vi "Autonomous Independent.vi"() -> ()   [LabVIEW 2020]
doc: "This VI is called when autonomous begins, and will automatically be terminated when autonomous ends. You can carry out timed or sensor driven robot movement independently without needing to return to the caller."
uses:
  <vilib>/Rock Robotics/WPI/ThirdParty/Phoenix-LabVIEW/Motor Controller/Controls/CTRE_Phoenix_MotorControl_ControlMode.ctl
  <vilib>/Rock Robotics/WPI/Solenoid/WPI_SolenoidValue.ctl
  <vilib>/Rock Robotics/WPI/Utilities/WPI_GetSetVariantRefNum.vi
  <vilib>/Rock Robotics/Network Tables/NT Read String.vi
  <vilib>/Rock Robotics/Network Tables/NT Write Numeric Array.vi
  <vilib>/Rock Robotics/WPI/Solenoid/WPI_SolenoidSetEnum.vi
  <vilib>/Rock Robotics/Network Tables/NT Read Number.vi
panel:
  out "Ty 22":dbl
  out "Ty 21":dbl
  out "Ty 20":dbl
  out "Ty 19":dbl
  out "Ty 18":dbl
  out "Ty 17":dbl
  out "Orange Limit Pressed 10":bool
  out "Blue Limit Pressed 10":bool
  out "Ty 16":dbl
  out "Orange Limit Pressed 9":bool
  out "Blue Limit Pressed 9":bool
  out "Ty 15":dbl
  out "Intake 5":bool
  out "Elevate 5":bool
  out "Ty 14":dbl
  out "Ty 13":dbl
  out "Ty 12":dbl
  out "Ty 11":dbl
  out "Ty 10":dbl
  out "Ty 9":dbl
  out "Orange Limit Pressed 4":bool
  out "Blue Limit Pressed 4":bool
  out "Ty 4":dbl
  out "Orange Limit Pressed 3":bool
  out "Blue Limit Pressed 3":bool
  out "Ty 3":dbl
  out "Intake 2":bool
  out "Elevate 2":bool
  out "Intake":bool
  out "Elevate":bool
  out "Orange Limit Pressed":bool
  out "Blue Limit Pressed":bool
  out "Ty":dbl
  out "Orange Limit Pressed 2":bool
  out "Blue Limit Pressed 2":bool
  out "Ty 2":dbl
  out "Intake 3":bool
  out "Elevate 3":bool
  out "Orange Limit Pressed 5":bool
  out "Blue Limit Pressed 5":bool
  out "Ty 5":dbl
  out "Orange Limit Pressed 6":bool
  out "Blue Limit Pressed 6":bool
  out "Ty 6":dbl
  out "Intake 4":bool
  out "Elevate 4":bool
  out "Orange Limit Pressed 7":bool
  out "Blue Limit Pressed 7":bool
  out "Ty 7":dbl
  out "Orange Limit Pressed 8":bool
  out "Blue Limit Pressed 8":bool
  out "Ty 8":dbl
  # "Be sure to right-click and choose Data Operations>>Make Current Value default if you want to save the array values with the VI"
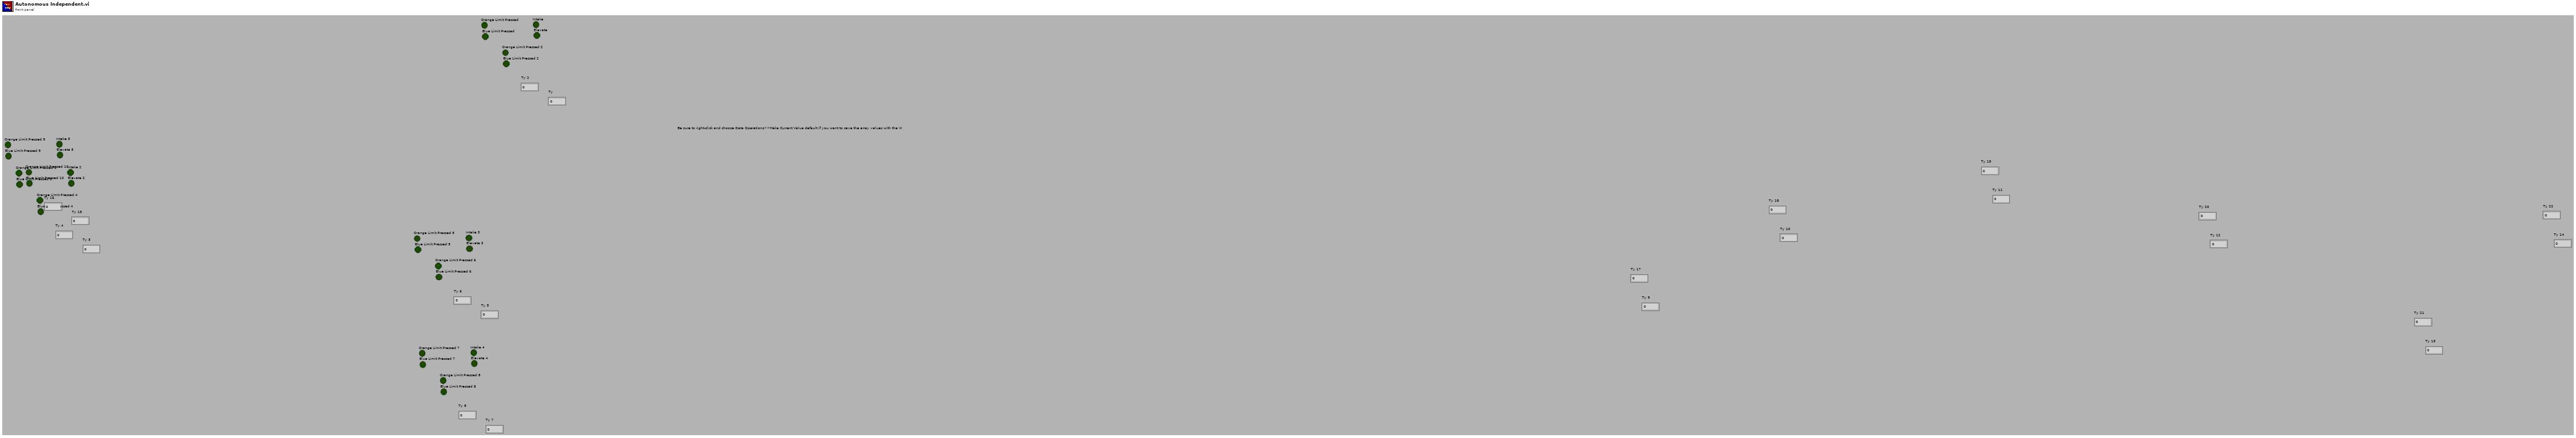
[diagram p1: front panel]
types:
  T1 = typedef "WPI_JoystickDevRef.ctl" = cluster{"Device":T2}
  T2 = typedef "WPI_JoystickDeviceEnum.ctl" = enum16{"USB 0", "USB 1", "USB 2", "USB 3", "USB 4", "USB 5"}
  T3 = typedef "WPI_SolenoidValue.ctl" = enum16{"Off", "On", "Forward", "Reverse"}
  T4 = typedef "WPI_SwitchDevRef.ctl" = cluster{"DevStatus":errorcluster, "DIO Channel":T5, "CntIndex":T6, "Normally Closed":bool}
  T5 = typedef "FPGA_DIOChannel.ctl" = enum8{"DIO 0", "DIO 1", "DIO 2", "DIO 3", "DIO 4", "DIO 5", "DIO 6", "DIO 7", "DIO 8", "DIO 9", "DIO MXP 0", "DIO MXP 1", "DIO MXP 2", "DIO MXP 3", "DIO MXP 4", "DIO MXP 5", "DIO MXP 6", "DIO MXP 7", "DIO MXP 8", "DIO MXP 9", "DIO MXP 10", "DIO MXP 11", "DIO MXP 12", "DIO MXP 13", "DIO MXP 14", "DIO MXP 15", "SPI Port CS1", "SPI Port CS2", "SPI Port CS3", "SPI Port MISO", "SPI Port MOSI", "Invalid"}
  T6 = typedef "FPGA_CounterCtrSystemIndex.ctl" = enum8{"Ctr 0", "Ctr 1", "Ctr 2", "Ctr 3", "Ctr 4", "Ctr 5", "Ctr 6", "Ctr 7", "Invalid"}
  T7 = typedef "WPI_SolenoidDevRef.ctl" = cluster{"DevStatus":errorcluster, "Pneumatics Control Module":u8, "Forward Solenoid Channel":T8, "Reverse Solenoid Channel":T8}
  T8 = typedef "WPI_SolenoidChannel.ctl" = enum8{"Solenoid 0", "Solenoid 1", "Solenoid 2", "Solenoid 3", "Solenoid 4", "Solenoid 5", "Solenoid 6", "Solenoid 7", "Solenoid 8", "Solenoid 9", "Solenoid 10", "Solenoid 11", "Solenoid 12", "Solenoid 13", "Solenoid 14", "Solenoid 15", "Invalid"}
  T9 = typedef "WPI_MotorControlDeviceRef.ctl" = cluster{"DeviceStatus":errorcluster, "Type":T10, "PWM":cluster{"PWM Channel":T11, "DeadBand":T12}, "CAN":cluster{"Device Number":u8, "SetOutput VI Ref":variant, "GetOutput VI Ref":variant, "Enable VI Ref":variant, "Disable VI Ref":variant, "Data":variant}, "Invert":bool, "DIO PWM":cluster{"PWM \"Enable\" Channel":T11, "DIOChannel":T5, "PWM Rate":dbl}}
  T10 = typedef "WPI_MotorControlType.ctl" = enum16{"PWM", "CAN", "DIO PWM"}
  T11 = typedef "FPGA_DIOPWMChannel.ctl" = enum8{"PWM 0", "PWM 1", "PWM 2", "PWM 3", "PWM 4", "PWM 5", "PWM 6", "PWM 7", "PWM 8", "PWM 9", "PWM MXP 0", "PWM MXP 1", "PWM MXP 2", "PWM MXP 3", "PWM MXP 4", "PWM MXP 5", "PWM MXP 6", "PWM MXP 7", "PWM MXP 8", "PWM MXP 9", "Invalid"}
  T12 = typedef "WPI_PWMDeadband.ctl" = cluster{"Name":string, "maxPositivePwm":i32, "minPositivePwm":i32, "centerPwm":i32, "maxNegativePwm":i32, "minNegativePwm":i32, "angularRange":u16}
  T13 = typedef "CTRE_Phoenix_MotorControl_ControlMode.ctl" = u16
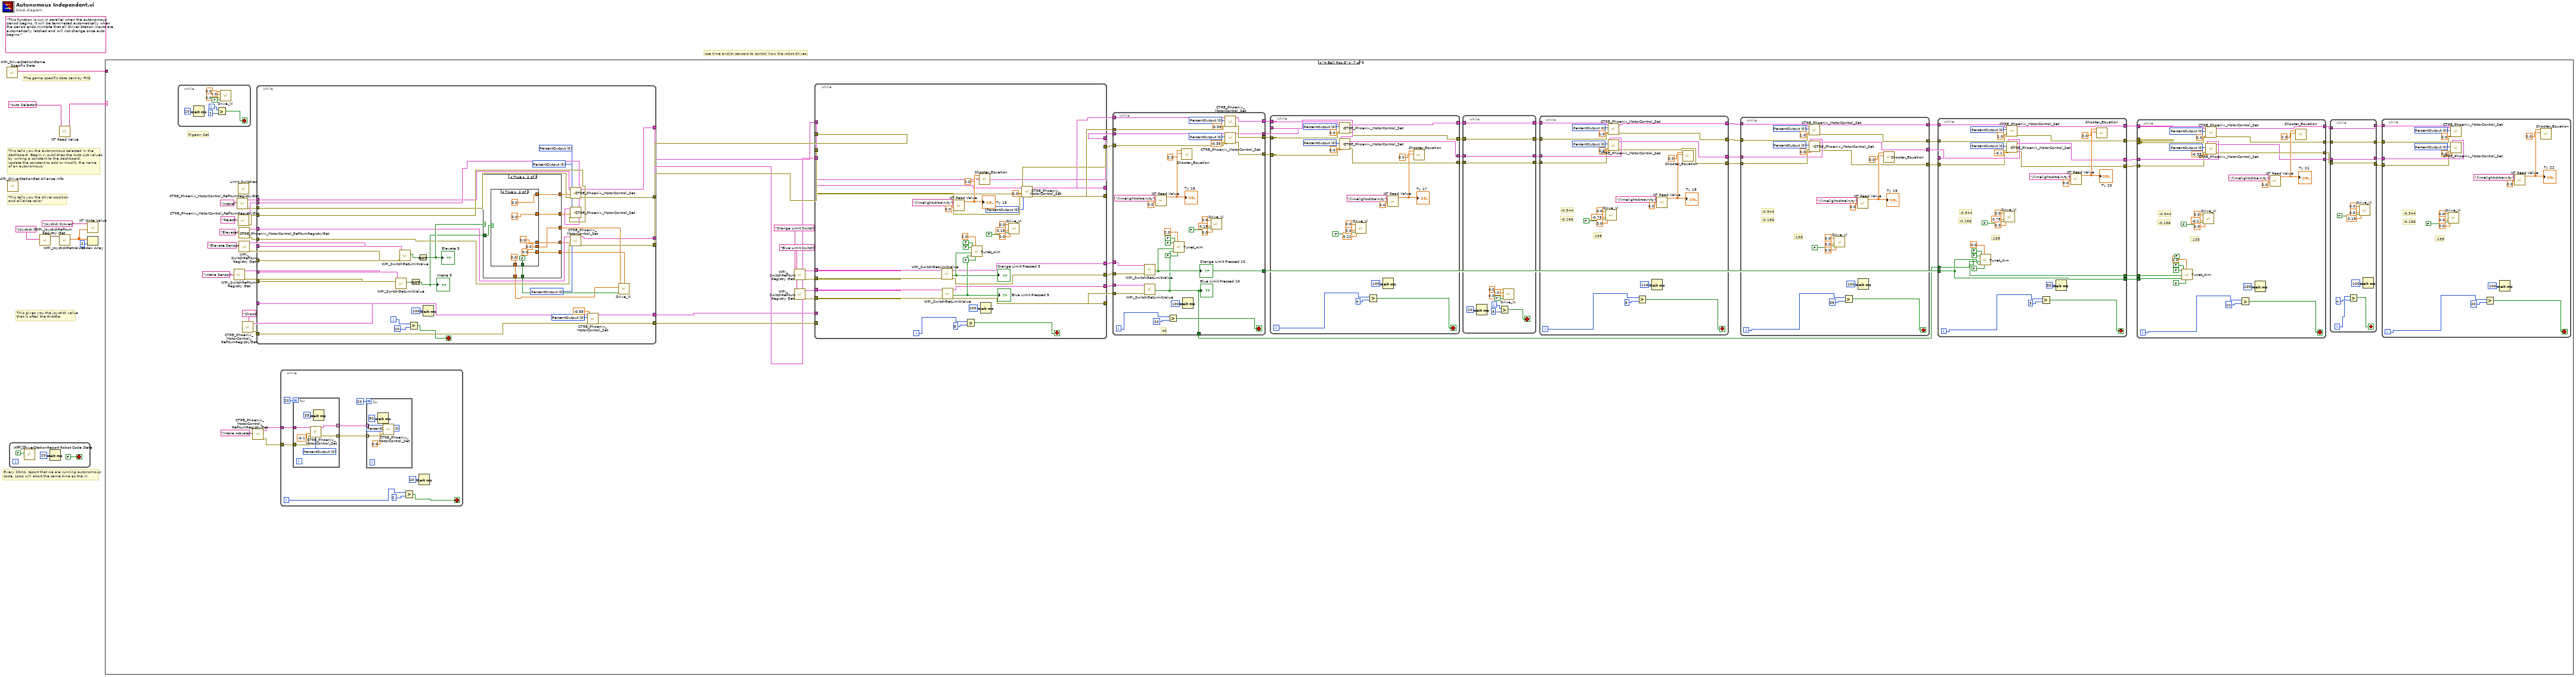
[diagram p0: block diagram]
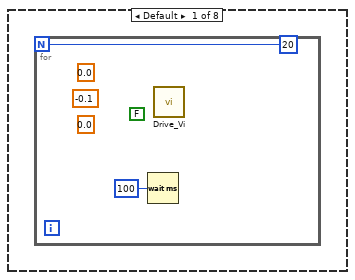
[diagram p2: hidden frame]
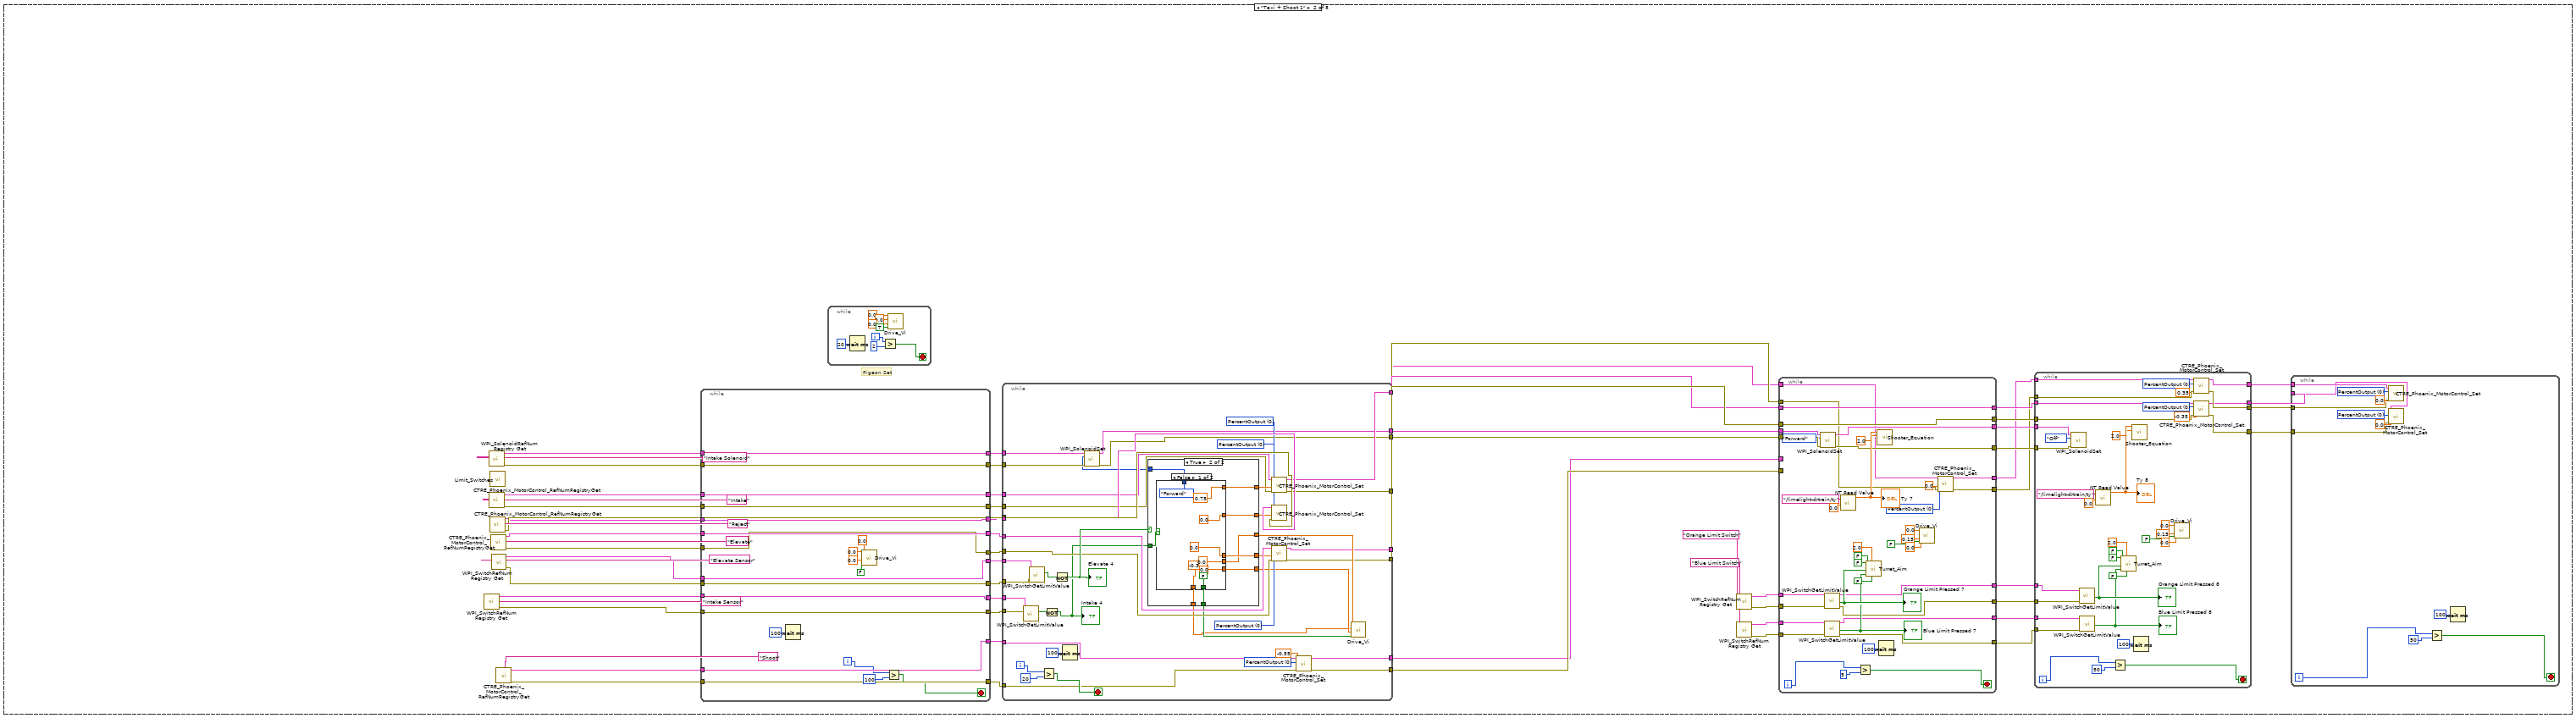
[diagram p3: hidden frame]
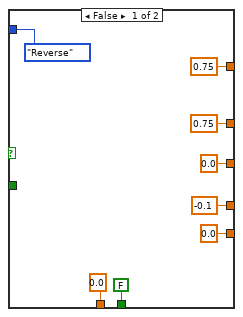
[diagram p4: hidden frame]
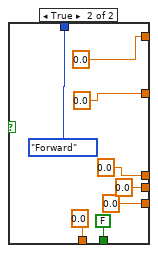
[diagram p5: hidden frame]
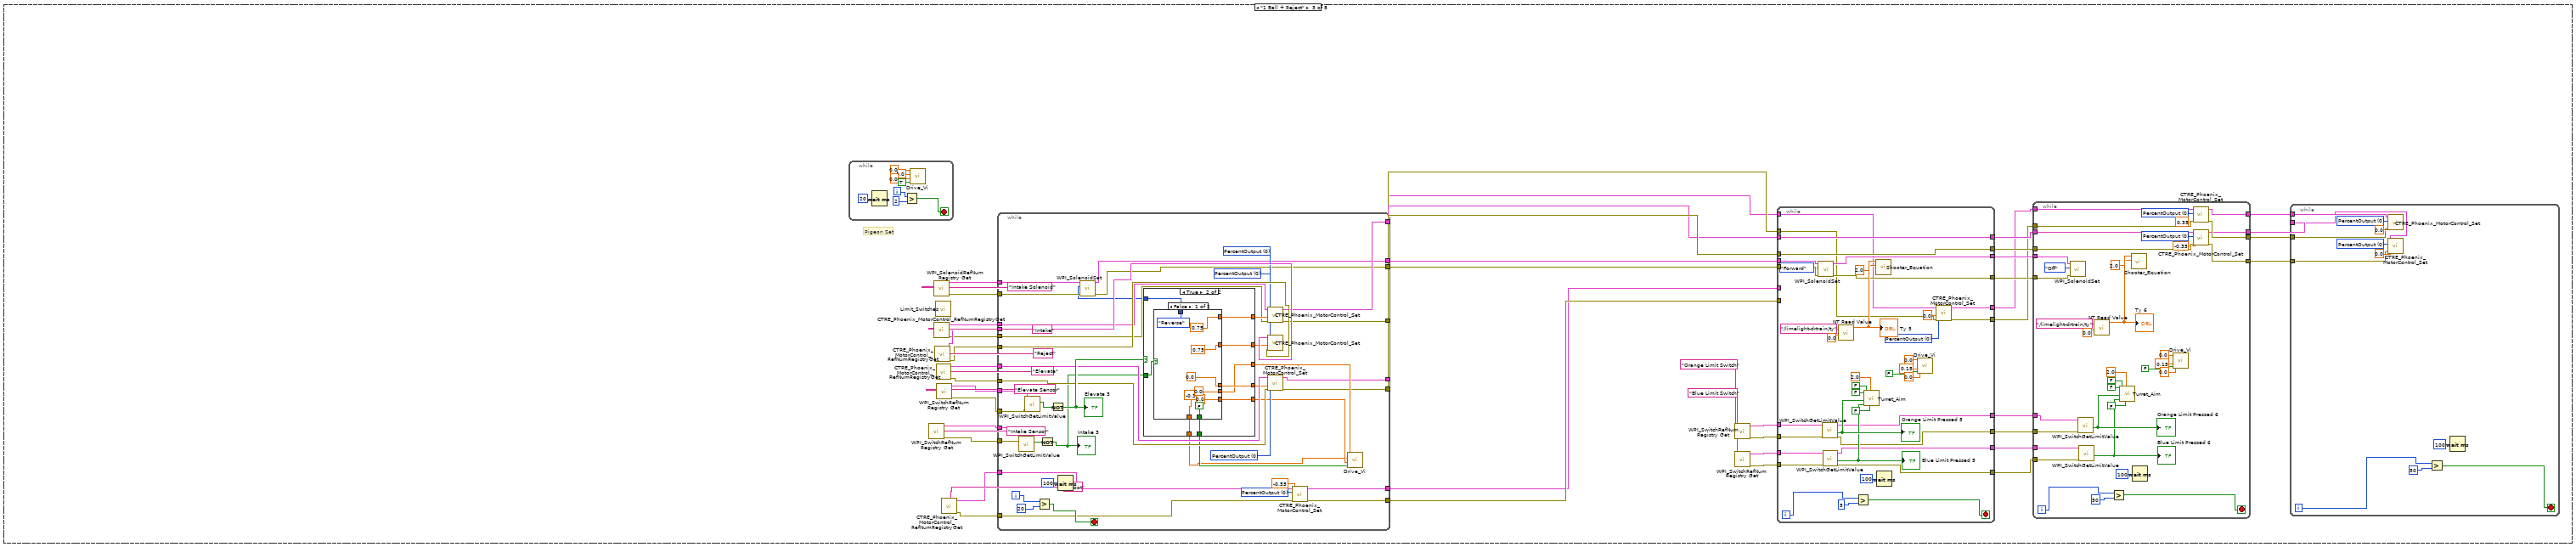
[diagram p6: hidden frame]
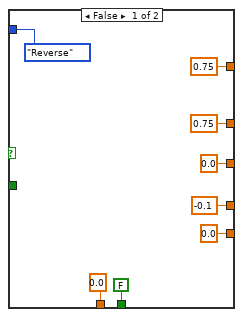
[diagram p7: hidden frame]
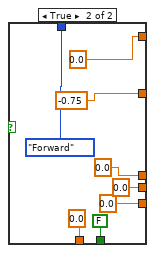
[diagram p8: hidden frame]
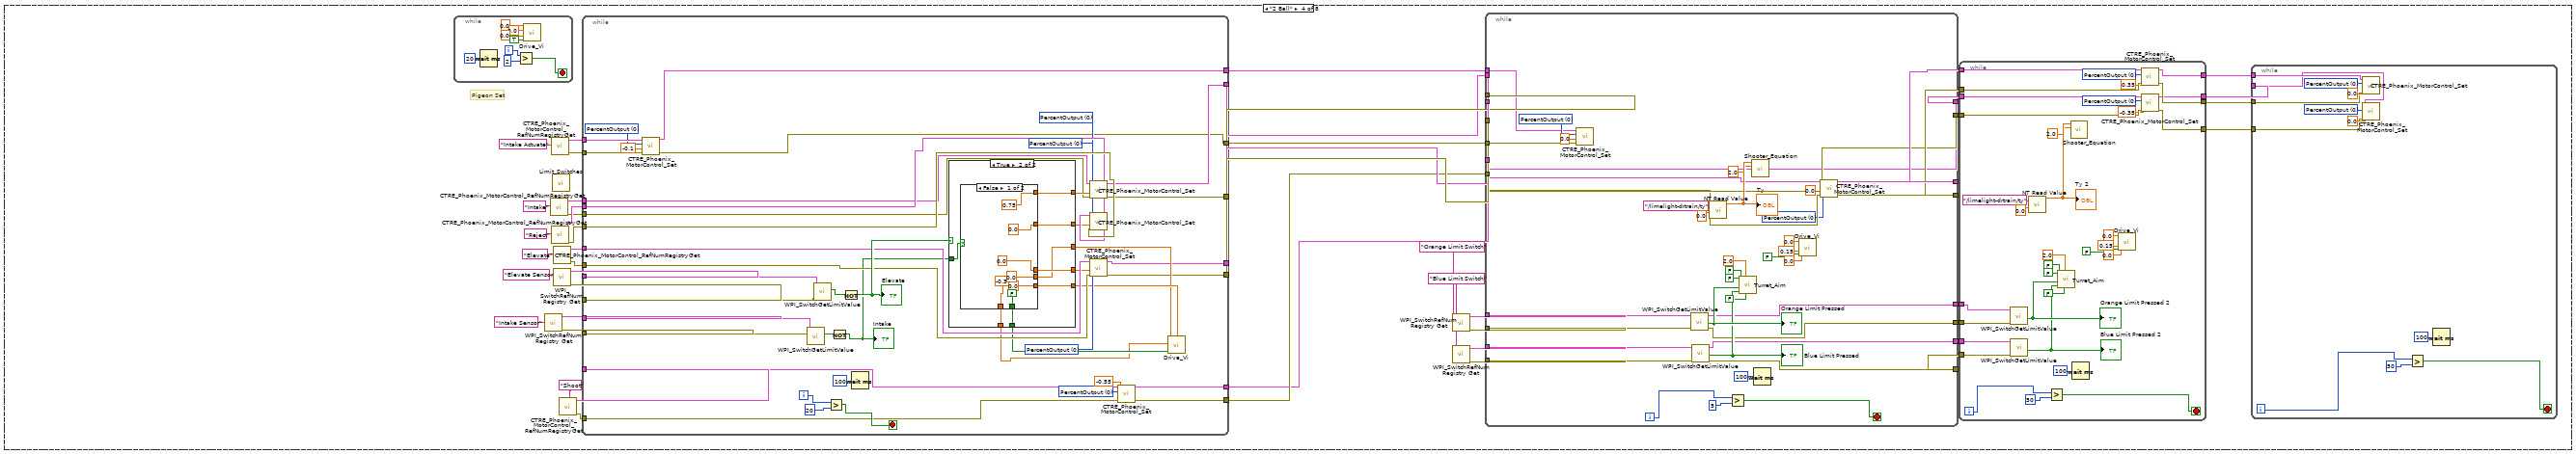
[diagram p9: hidden frame]
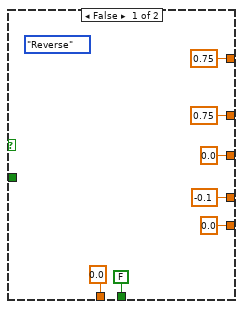
[diagram p10: hidden frame]
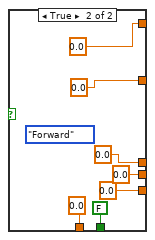
[diagram p11: hidden frame]
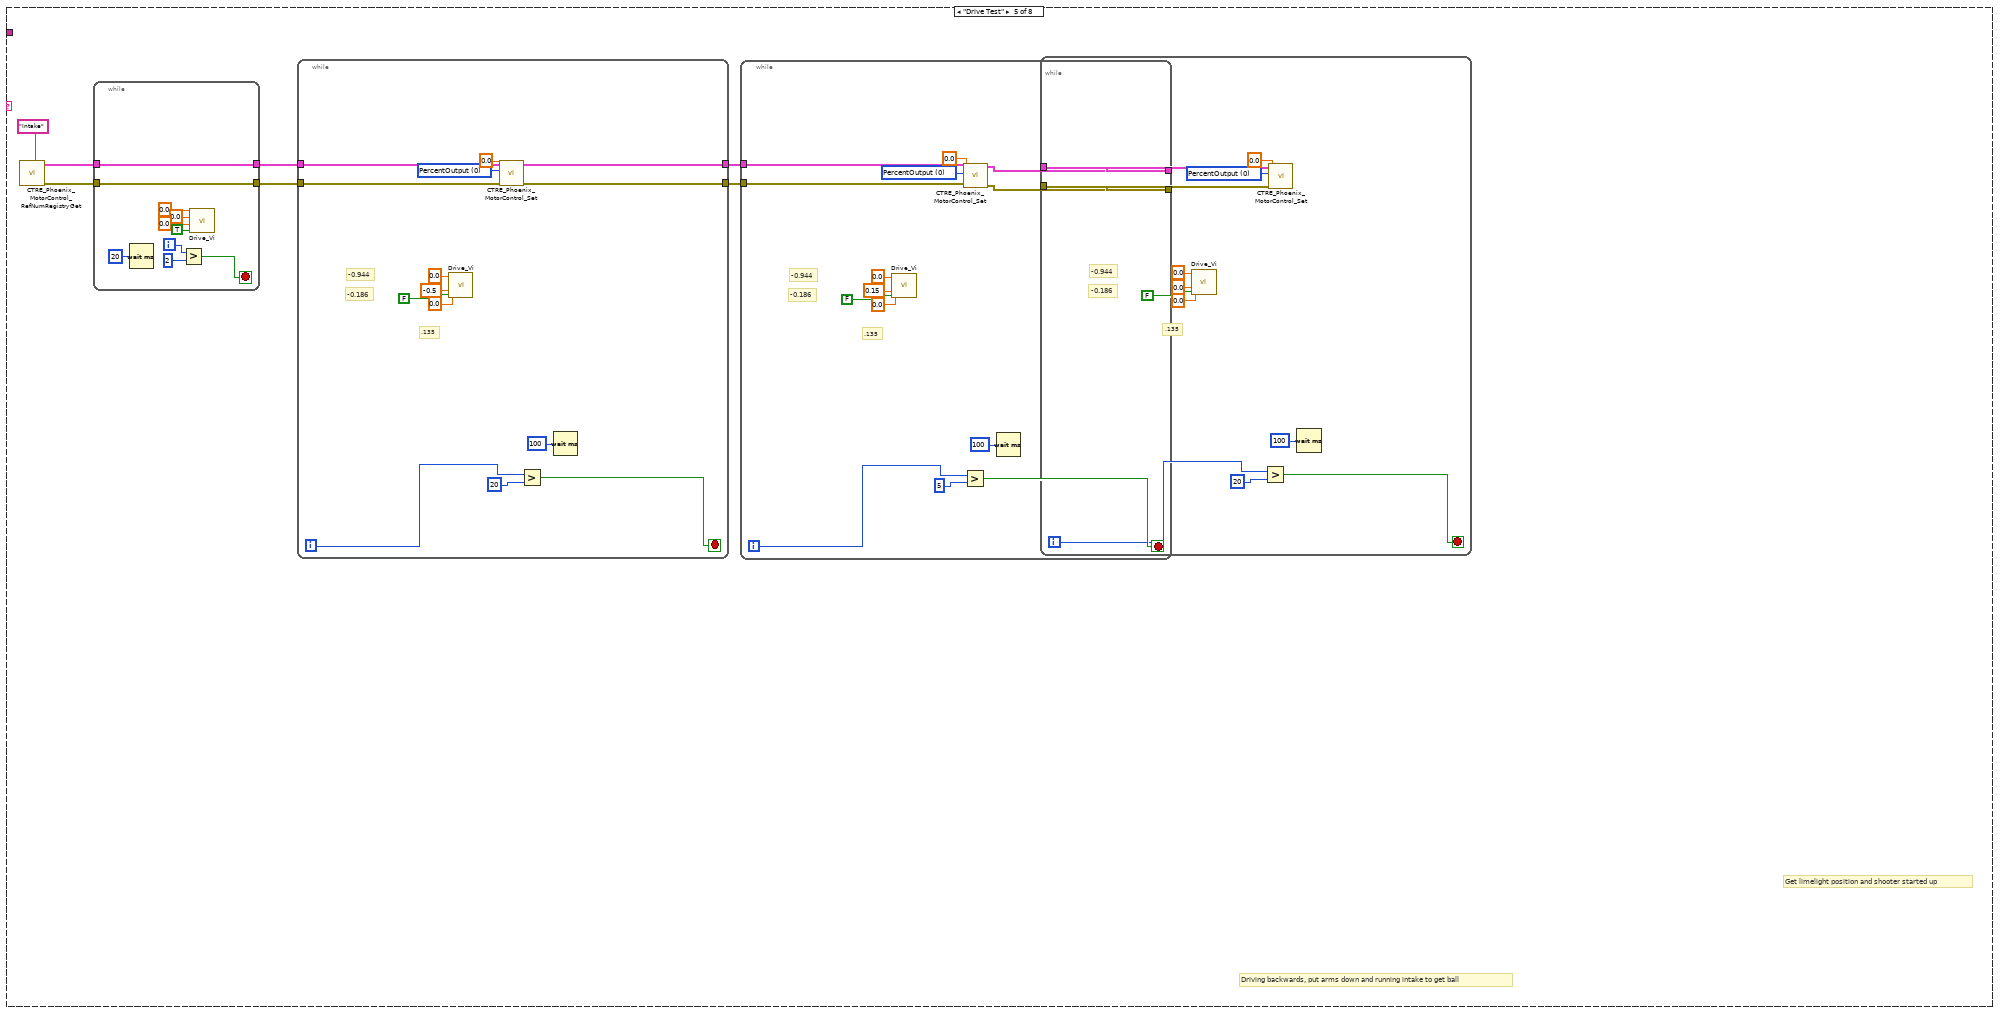
[diagram p12: hidden frame]
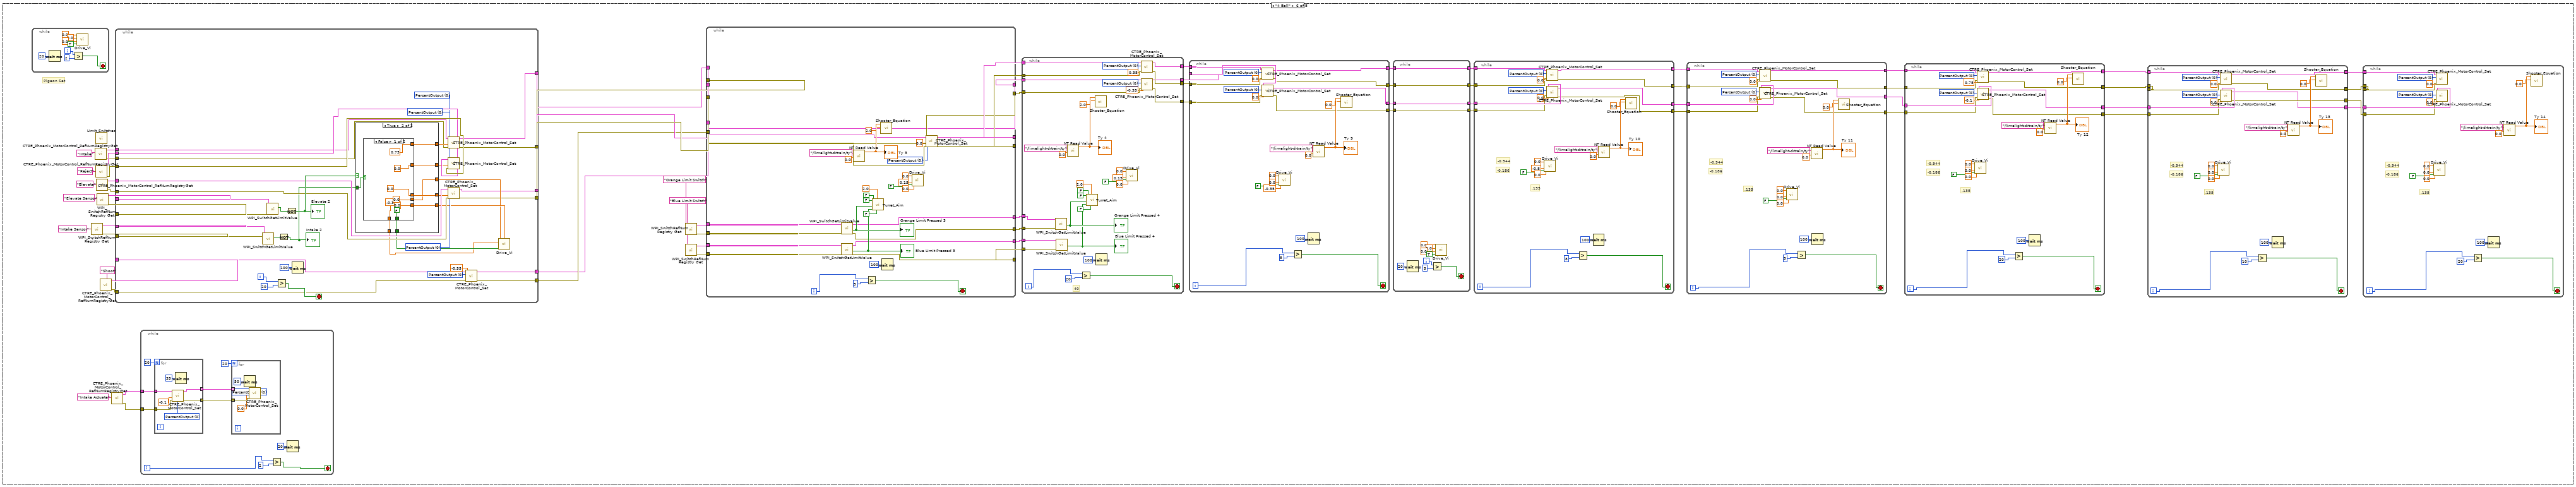
[diagram p13: hidden frame]
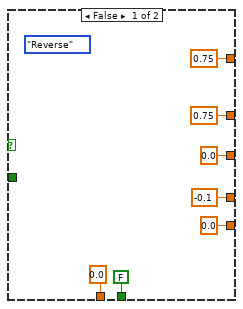
[diagram p14: hidden frame]
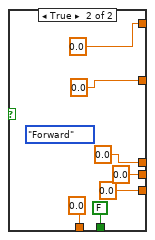
[diagram p15: hidden frame]
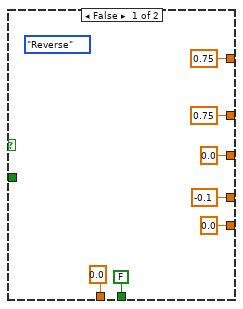
[diagram p16: hidden frame]
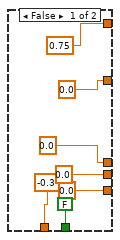
[diagram p17: hidden frame]
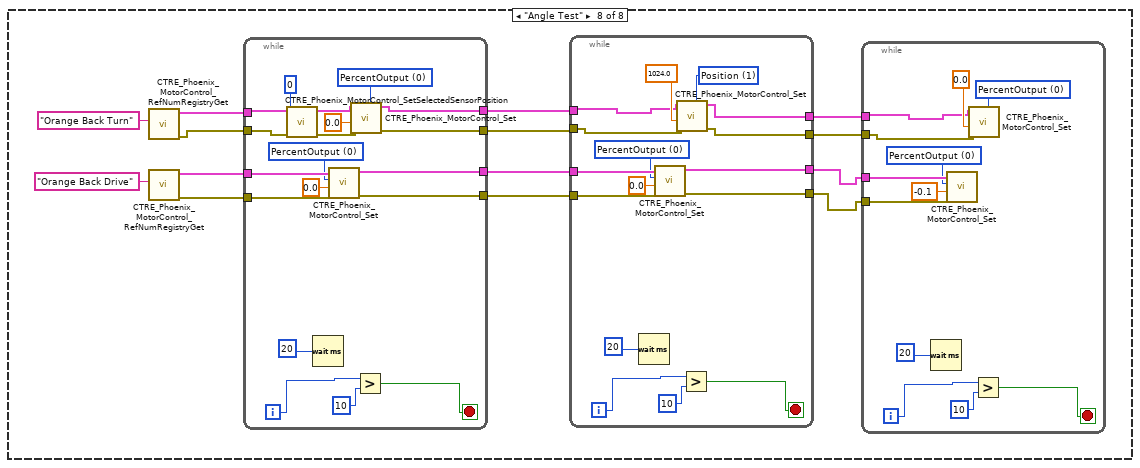
[diagram p18: hidden frame]
diagram:
  (unwired) "This function is run in parallel when the autonomous period begins. It will be terminated automatically when the period ends.\n\nNote that all Driver Station inputs are automatically latched and will not change once auto begins."
  # "The game specific data sent by FMS"
  # "This tells you the autonomous selected in the \ndashboard. Begin.vi publishes the Auto List values\nby writing a constant to the dashboard.\nUpdate the constant to add or modify the name\nof an autonomous."
  # "Every 20ms, report that we are running autonomous\ncode. Loop will abort the same time as the VI."
  # "This gives you the joystick value\nthat is often the throttle"
  # "Use time and/or sensors to control how the robot drives."
  # "This tells you the driver position\nand alliance color"
  n1 = call <vilib>:"WPI_DriverStationGame Specific Data.vi"() -> ("Game Specific Data"=w1:string)  [unwired: 11 in]
  n2 = call <vilib>:"WPI_DriverStationGet Alliance Info.vi"() -> ()  [unwired: 12 out]
  n3 = while {
    stop <- FALSE stop-if-true
    n4 = call <vilib>:"WPI_DriverStationReport Robot Code State.vi"("Autonomous"=TRUE) -> ()  [unwired: 10 in, 1 out]
    n5 = Wait (ms)(milliseconds to wait=u32 20) -> ()  [unwired: 1 out]
  }
  n6 = call <vilib>:"WPI_JoystickRefNum Registry Get.vi"("refnum name"="Joystick 0") -> ("JoystickDevRef"=w7:T1)  [unwired: 1 in, 9 out]
  n7 = call <vilib>:"WPI_JoystickGetValues.vi"("JoystickDevRef"=w7) -> ("Axes"=w3:dbl[])  [unwired: 6 in, 4 out]
  n8 = call-poly <vilib>:"NT Read Value.vi"("Name"="Auto Selector") -> ("String"=w4:string)  [unwired: 9 in, 1 out]
  n9 = call-poly <vilib>:"NT Write Value.vi"("Numeric Array"=w3, "Name"="Joystick 0/Axes") -> ()  [unwired: 9 in, 1 out]
  n10 = Index Array(array=w3, index=2) -> ()  [unwired: 1 out]
  n11 = case shown="\"4 Ball Pos 3\"" w4 {
    tunnel: w1 -> [_ _ _ _ _ _ _ _]
    frame Default {
      n12 = for {
        N: 20 -> [_]
        (unwired) FALSE ("Middle Thumb")
        (unwired) 0.0 ("Z")
        (unwired) -0.1 ("Y")
        (unwired) 0.0 ("X")
        n13 = Wait (ms)(milliseconds to wait=u32 100) -> ()  [unwired: 1 out]
        n14 = call "Drive_Vi.vi"() -> ()  [unwired: 12 in]
      }
    }
    frame "Taxi + Shoot 1" {
      # "Pigeon Set"
      n15 = call <vilib>:"WPI_SwitchRefNum Registry Get.vi"("refnum name"="Intake Sensor") -> ("error out"=w18:errorcluster, "SwitchDevRef"=w20:T4)  [unwired: 9 in]
      n16 = call <vilib>:"WPI_SolenoidRefNum Registry Get.vi"("refnum name"="Intake Solenoid") -> ("error out"=w37:errorcluster, "SolenoidDevRef"=w39:T7)  [unwired: 9 in]
      n17 = call <vilib>:"CTRE_Phoenix_MotorControl_RefNumRegistryGet.vi"("refnum name"="Intake") -> ("error out"=w32:errorcluster, "PhoenixMotorControlDevRef"=w34:T9)  [unwired: 9 in]
      n18 = call <vilib>:"CTRE_Phoenix_MotorControl_RefNumRegistryGet.vi"("refnum name"="Reject") -> ("error out"=w68:errorcluster, "PhoenixMotorControlDevRef"=w30:T9)  [unwired: 9 in]
      n19 = call "Limit_Switches.vi"() -> ()  [unwired: 10 in, 2 out]
      n20 = call <vilib>:"CTRE_Phoenix_MotorControl_RefNumRegistryGet.vi"("refnum name"="Elevate") -> ("error out"=w26:errorcluster, "PhoenixMotorControlDevRef"=w28:T9)  [unwired: 9 in]
      n21 = call <vilib>:"WPI_SwitchRefNum Registry Get.vi"("refnum name"="Elevate Sensor") -> ("error out"=w22:errorcluster, "SwitchDevRef"=w24:T4)  [unwired: 9 in]
      n22 = call <vilib>:"CTRE_Phoenix_MotorControl_RefNumRegistryGet.vi"("refnum name"="Shoot") -> ("error out"=w14:errorcluster, "PhoenixMotorControlDevRef"=w17:T9)  [unwired: 9 in]
      n23 = while {
        tunnel: [w92] -> w38
        tunnel: w39 -> [w92]
        tunnel: [w91] -> w36
        tunnel: w37 -> [w91]
        tunnel: [w90] -> w35
        tunnel: w34 -> [w90]
        tunnel: [w89] -> w33
        tunnel: w32 -> [w89]
        tunnel: [w88] -> w31
        tunnel: w30 -> [w88]
        tunnel: [w87] -> w29
        tunnel: w28 -> [w87]
        tunnel: [w86] -> w27
        tunnel: w26 -> [w86]
        tunnel: [w85] -> w25
        tunnel: w24 -> [w85]
        tunnel: [w84] -> w23
        tunnel: w22 -> [w84]
        tunnel: [w83] -> w21
        tunnel: w20 -> [w83]
        tunnel: [w82] -> w19
        tunnel: w18 -> [w82]
        tunnel: [w81] -> w16
        tunnel: w17 -> [w81]
        tunnel: [w80] -> w15
        tunnel: w14 -> [w80]
        i -> [w76]
        stop <- w78 stop-if-true
        n24 = Wait (ms)(milliseconds to wait=u32 100) -> ()  [unwired: 1 out]
        n25 = call "Drive_Vi.vi"("Middle Thumb"=FALSE, "Z"=0.0, "Y"=0.0, "X"=0.0) -> ()  [unwired: 8 in]
        n26 = Greater?(x=w76, y=100) -> (0:w78:bool)
      }
      n27 = while {
        i -> [w266]
        stop <- w267 stop-if-true
        n28 = Wait (ms)(milliseconds to wait=u32 20) -> ()  [unwired: 1 out]
        n29 = Greater?(x=w266, y=2) -> (0:w267:bool)
        n30 = call "Drive_Vi.vi"("Middle Thumb"=TRUE, "Z"=0.0, "Y"=0.0, "X"=0.0) -> ()  [unwired: 8 in]
      }
      n31 = while {
        tunnel: w23 -> [w221]
        tunnel: w25 -> [w220]
        tunnel: w19 -> [w219]
        tunnel: w21 -> [w218]
        tunnel: w36 -> [w217]
        tunnel: w38 -> [w216]
        tunnel: w27 -> [w213]
        tunnel: w29 -> [w212]
        tunnel: w68 -> [w211]
        tunnel: w31 -> [w210]
        tunnel: w33 -> [w209]
        tunnel: w35 -> [w208]
        tunnel: [w196] -> w61
        tunnel: [w195] -> w60
        tunnel: [w194] -> w59
        tunnel: [w193] -> w58
        tunnel: w15 -> [w192]
        tunnel: w16 -> [w191]
        tunnel: [w188] -> w57
        tunnel: [w187] -> w56
        tunnel: [w186] -> w49
        tunnel: [w185] -> w48
        i -> [w224]
        stop <- w225 stop-if-true
        w190 = T13 0 items=["PercentOutput"=0, "Position"=1, "Velocity"=2, "Current"=3, "Follower"=5, "MotionProfile"=6, "MotionMagic"=7, "MotionProfileArc"=10, "Disabled"=15] ("Control Mode")
        w202 = T13 0 items=["PercentOutput"=0, "Position"=1, "Velocity"=2, "Current"=3, "Follower"=5, "MotionProfile"=6, "MotionMagic"=7, "MotionProfileArc"=10, "Disabled"=15] ("Control Mode")
        w203 = T13 0 items=["PercentOutput"=0, "Position"=1, "Velocity"=2, "Current"=3, "Follower"=5, "MotionProfile"=6, "MotionMagic"=7, "MotionProfileArc"=10, "Disabled"=15] ("Control Mode")
        w204 = T13 0 items=["PercentOutput"=0, "Position"=1, "Velocity"=2, "Current"=3, "Follower"=5, "MotionProfile"=6, "MotionMagic"=7, "MotionProfileArc"=10, "Disabled"=15] ("Control Mode")
        n32 = call <vilib>:"WPI_SwitchGetLimitValue.vi"("error in (no error)"=w219, "SwitchDevRef"=w218) -> ("Switch Pressed"=w222:bool)  [unwired: 7 in, 2 out]
        n33 = call <vilib>:"WPI_SwitchGetLimitValue.vi"("error in (no error)"=w221, "SwitchDevRef"=w220) -> ("Switch Pressed"=w223:bool)  [unwired: 7 in, 2 out]
        n34 = Greater?(x=w224, y=20) -> (0:w225:bool)
        n35 = Not(x=w222) -> (.not. x?=w207:bool)
        "Intake 4" <- w207
        n36 = Not(x=w223) -> (.not. x?=w215:bool)
        "Elevate 4" <- w215
        n37 = Wait (ms)(milliseconds to wait=u32 100) -> ()  [unwired: 1 out]
        n38 = case shown="True" w215 {
          tunnel: [0.75 ("Output") w244] -> w214
          tunnel: w207 -> [_ w241]
          tunnel: [0.75 ("Output") w243] -> w206
          tunnel: [-0.1 ("Output") w242] -> w205
          tunnel: [FALSE ("Middle Thumb") w240] -> w201
          tunnel: [0.0 ("Z") w239] -> w200
          tunnel: [0.0 ("Y") w238] -> w199
          tunnel: [0.0 ("X") w237] -> w198
          tunnel: [WPI_SolenoidValue."Reverse" ("Value") w236] -> w197
          frame False {
          }
          frame True {
            n39 = case shown="False" w241 {
              tunnel: [0.75 ("Output") 0.0 ("Output")] -> w244
              tunnel: [0.0 ("Output") 0.0 ("Output")] -> w243
              tunnel: [0.0 ("Output") 0.0 ("Output")] -> w242
              tunnel: [FALSE ("Middle Thumb") FALSE ("Middle Thumb")] -> w240
              tunnel: [0.0 ("Z") 0.0 ("Z")] -> w239
              tunnel: [-0.3 ("Y") 0.0 ("Y")] -> w238
              tunnel: [0.0 ("X") 0.0 ("X")] -> w237
              tunnel: [WPI_SolenoidValue."Forward" ("Value") WPI_SolenoidValue."Forward" ("Value")] -> w236
              frame False {
              }
              frame True {
              }
            }
          }
        }
        n40 = call-poly <vilib>:"WPI_SolenoidSet.vi"("error in (no error)"=w217, "Value"=w197, "SolenoidDevRef"=w216) -> ("error out"=w185:errorcluster, "SolenoidDevRef"=w186:T7)  [unwired: 7 in]
        n41 = call <vilib>:"CTRE_Phoenix_MotorControl_Set.vi"("error in (no error)"=w209, "Output"=w214, "Control Mode"=w202, "PhoenixMotorControlDevRef"=w208) -> ("error out"=w194:errorcluster, "PhoenixMotorControlDevRef"=w193:T9)  [unwired: 6 in]
        n42 = call <vilib>:"CTRE_Phoenix_MotorControl_Set.vi"("error in (no error)"=w211, "Output"=w206, "Control Mode"=w203, "PhoenixMotorControlDevRef"=w210) -> ()  [unwired: 6 in, 2 out]
        n43 = call <vilib>:"CTRE_Phoenix_MotorControl_Set.vi"("error in (no error)"=w213, "Output"=w205, "Control Mode"=w204, "PhoenixMotorControlDevRef"=w212) -> ("error out"=w196:errorcluster, "PhoenixMotorControlDevRef"=w195:T9)  [unwired: 6 in]
        n44 = call <vilib>:"CTRE_Phoenix_MotorControl_Set.vi"("error in (no error)"=w192, "Output"=-0.55, "Control Mode"=w190, "PhoenixMotorControlDevRef"=w191) -> ("error out"=w188:errorcluster, "PhoenixMotorControlDevRef"=w187:T9)  [unwired: 6 in]
        n45 = call "Drive_Vi.vi"("Middle Thumb"=w201, "Z"=w200, "Y"=w199, "X"=w198) -> ()  [unwired: 8 in]
      }
      n46 = call <vilib>:"WPI_SwitchRefNum Registry Get.vi"("refnum name"="Orange Limit Switch") -> ("error out"=w63:errorcluster, "SwitchDevRef"=w62:T4)  [unwired: 9 in]
      n47 = call <vilib>:"WPI_SwitchRefNum Registry Get.vi"("refnum name"="Blue Limit Switch") -> ("error out"=w65:errorcluster, "SwitchDevRef"=w64:T4)  [unwired: 9 in]
      n48 = while {
        tunnel: w57 -> [_]
        tunnel: w56 -> [_]
        tunnel: w65 -> [w182]
        tunnel: w64 -> [w181]
        tunnel: w63 -> [w180]
        tunnel: w62 -> [w179]
        tunnel: w61 -> [w158]
        tunnel: w60 -> [w157]
        tunnel: w59 -> [w148]
        tunnel: w58 -> [w149]
        tunnel: [w162] -> w55
        tunnel: [w161] -> w54
        tunnel: [w160] -> w53
        tunnel: [w159] -> w52
        tunnel: [w158] -> w51
        tunnel: [w157] -> w50
        tunnel: w49 -> [w156]
        tunnel: w48 -> [w155]
        tunnel: [w153] -> w47
        tunnel: [w152] -> w46
        tunnel: [w151] -> w45
        tunnel: [w150] -> w44
        i -> [w168]
        stop <- w167 stop-if-true
        w147 = T13 0 items=["PercentOutput"=0, "Position"=1, "Velocity"=2, "Current"=3, "Follower"=5, "MotionProfile"=6, "MotionMagic"=7, "MotionProfileArc"=10, "Disabled"=15] ("Control Mode")
        n49 = call-poly <vilib>:"WPI_SolenoidSet.vi"("error in (no error)"=w155, "Value"=WPI_SolenoidValue."Forward", "SolenoidDevRef"=w156) -> ("error out"=w152:errorcluster, "SolenoidDevRef"=w153:T7)  [unwired: 7 in]
        n50 = call <vilib>:"WPI_SwitchGetLimitValue.vi"("error in (no error)"=w180, "SwitchDevRef"=w179) -> ("error out"=w159:errorcluster, "Switch Pressed"=w178:bool, "SwitchDevRef"=w160:T4)  [unwired: 7 in]
        "Orange Limit Pressed 7" <- w178
        n51 = call <vilib>:"WPI_SwitchGetLimitValue.vi"("error in (no error)"=w182, "SwitchDevRef"=w181) -> ("error out"=w161:errorcluster, "Switch Pressed"=w177:bool, "SwitchDevRef"=w162:T4)  [unwired: 7 in]
        "Blue Limit Pressed 7" <- w177
        n52 = call-poly <vilib>:"NT Read Value.vi"("Default Value"=0.0, "Name"="/limelight-drtrain/ty") -> ("Numeric"=w172:dbl)  [unwired: 8 in, 1 out]
        "Ty 7" <- w172
        n53 = Greater?(x=w168, y=5) -> (0:w167:bool)
        n54 = call "Turret_Aim.vi"("View Button"=FALSE ("Driver Right Thumb"), "Left Trigger"=2.0, "Orange Limit Pressed"=w177, "Blue Limit Pressed"=w178, "Right Bumper"=FALSE, "Left Bumper"=FALSE) -> ()  [unwired: 6 in]
        n55 = call "Shooter_Equation.vi"("Right Trigger"=2.0, "Ty"=w172) -> ()  [unwired: 10 in]
        n56 = Wait (ms)(milliseconds to wait=u32 100) -> ()  [unwired: 1 out]
        n57 = call "Drive_Vi.vi"("Middle Thumb"=FALSE, "Z"=0.0, "Y"=0.15, "X"=0.0) -> ()  [unwired: 8 in]
        n58 = call <vilib>:"CTRE_Phoenix_MotorControl_Set.vi"("error in (no error)"=w148, "Output"=0.0, "Control Mode"=w147, "PhoenixMotorControlDevRef"=w149) -> ("error out"=w150:errorcluster, "PhoenixMotorControlDevRef"=w151:T9)  [unwired: 6 in]
      }
      n59 = while {
        tunnel: w54 -> [w143]
        tunnel: w55 -> [w142]
        tunnel: w52 -> [w141]
        tunnel: w51 -> [w128]
        tunnel: w50 -> [w127]
        tunnel: w44 -> [w126]
        tunnel: w45 -> [w125]
        tunnel: w53 -> [w116]
        tunnel: w47 -> [w115]
        tunnel: w46 -> [w114]
        tunnel: [w112] -> w43
        tunnel: [w111] -> w42
        tunnel: [w110] -> w41
        tunnel: [w109] -> w40
        i -> [w130]
        stop <- w129 stop-if-true
        w123 = T13 0 items=["PercentOutput"=0, "Position"=1, "Velocity"=2, "Current"=3, "Follower"=5, "MotionProfile"=6, "MotionMagic"=7, "MotionProfileArc"=10, "Disabled"=15] ("Control Mode")
        w124 = T13 0 items=["PercentOutput"=0, "Position"=1, "Velocity"=2, "Current"=3, "Follower"=5, "MotionProfile"=6, "MotionMagic"=7, "MotionProfileArc"=10, "Disabled"=15] ("Control Mode")
        n60 = call-poly <vilib>:"WPI_SolenoidSet.vi"("error in (no error)"=w114, "Value"=WPI_SolenoidValue."Off", "SolenoidDevRef"=w115) -> ()  [unwired: 7 in, 2 out]
        n61 = call <vilib>:"WPI_SwitchGetLimitValue.vi"("error in (no error)"=w141, "SwitchDevRef"=w116) -> ("Switch Pressed"=w140:bool)  [unwired: 7 in, 2 out]
        "Orange Limit Pressed 8" <- w140
        n62 = call <vilib>:"WPI_SwitchGetLimitValue.vi"("error in (no error)"=w143, "SwitchDevRef"=w142) -> ("Switch Pressed"=w139:bool)  [unwired: 7 in, 2 out]
        "Blue Limit Pressed 8" <- w139
        n63 = call-poly <vilib>:"NT Read Value.vi"("Default Value"=0.0, "Name"="/limelight-drtrain/ty") -> ("Numeric"=w134:dbl)  [unwired: 8 in, 1 out]
        "Ty 8" <- w134
        n64 = Greater?(x=w130, y=50) -> (0:w129:bool)
        n65 = call "Turret_Aim.vi"("View Button"=FALSE ("Driver Right Thumb"), "Left Trigger"=2.0, "Orange Limit Pressed"=w139, "Blue Limit Pressed"=w140, "Right Bumper"=FALSE, "Left Bumper"=FALSE) -> ()  [unwired: 6 in]
        n66 = call "Shooter_Equation.vi"("Right Trigger"=2.0, "Ty"=w134) -> ()  [unwired: 10 in]
        n67 = Wait (ms)(milliseconds to wait=u32 100) -> ()  [unwired: 1 out]
        n68 = call "Drive_Vi.vi"("Middle Thumb"=FALSE, "Z"=0.0, "Y"=0.15, "X"=0.0) -> ()  [unwired: 8 in]
        n69 = call <vilib>:"CTRE_Phoenix_MotorControl_Set.vi"("error in (no error)"=w126, "Output"=0.35, "Control Mode"=w123, "PhoenixMotorControlDevRef"=w125) -> ("error out"=w112:errorcluster, "PhoenixMotorControlDevRef"=w111:T9)  [unwired: 6 in]
        n70 = call <vilib>:"CTRE_Phoenix_MotorControl_Set.vi"("error in (no error)"=w128, "Output"=-0.35, "Control Mode"=w124, "PhoenixMotorControlDevRef"=w127) -> ("error out"=w109:errorcluster, "PhoenixMotorControlDevRef"=w110:T9)  [unwired: 6 in]
      }
      n71 = while {
        tunnel: w43 -> [w104]
        tunnel: w42 -> [w103]
        tunnel: w41 -> [w102]
        tunnel: w40 -> [w101]
        i -> [w99]
        stop <- w98 stop-if-true
        w107 = T13 0 items=["PercentOutput"=0, "Position"=1, "Velocity"=2, "Current"=3, "Follower"=5, "MotionProfile"=6, "MotionMagic"=7, "MotionProfileArc"=10, "Disabled"=15] ("Control Mode")
        w108 = T13 0 items=["PercentOutput"=0, "Position"=1, "Velocity"=2, "Current"=3, "Follower"=5, "MotionProfile"=6, "MotionMagic"=7, "MotionProfileArc"=10, "Disabled"=15] ("Control Mode")
        n72 = call <vilib>:"CTRE_Phoenix_MotorControl_Set.vi"("error in (no error)"=w104, "Output"=0.0, "Control Mode"=w107, "PhoenixMotorControlDevRef"=w103) -> ()  [unwired: 6 in, 2 out]
        n73 = call <vilib>:"CTRE_Phoenix_MotorControl_Set.vi"("error in (no error)"=w101, "Output"=0.0, "Control Mode"=w108, "PhoenixMotorControlDevRef"=w102) -> ()  [unwired: 6 in, 2 out]
        n74 = Greater?(x=w99, y=50) -> (0:w98:bool)
        n75 = Wait (ms)(milliseconds to wait=u32 100) -> ()  [unwired: 1 out]
      }
    }
    frame "1 Ball + Reject" {
      # "Pigeon Set"
      n76 = while {
        i -> [w487]
        stop <- w488 stop-if-true
        n77 = Wait (ms)(milliseconds to wait=u32 20) -> ()  [unwired: 1 out]
        n78 = Greater?(x=w487, y=2) -> (0:w488:bool)
        n79 = call "Drive_Vi.vi"("Middle Thumb"=TRUE, "Z"=0.0, "Y"=0.0, "X"=0.0) -> ()  [unwired: 8 in]
      }
      n80 = call <vilib>:"WPI_SwitchRefNum Registry Get.vi"("refnum name"="Intake Sensor") -> ("error out"=w308:errorcluster, "SwitchDevRef"=w307:T4)  [unwired: 9 in]
      n81 = call <vilib>:"WPI_SolenoidRefNum Registry Get.vi"("refnum name"="Intake Solenoid") -> ("error out"=w306:errorcluster, "SolenoidDevRef"=w305:T7)  [unwired: 9 in]
      n82 = call <vilib>:"CTRE_Phoenix_MotorControl_RefNumRegistryGet.vi"("refnum name"="Intake") -> ("error out"=w300:errorcluster, "PhoenixMotorControlDevRef"=w299:T9)  [unwired: 9 in]
      n83 = call <vilib>:"CTRE_Phoenix_MotorControl_RefNumRegistryGet.vi"("refnum name"="Reject") -> ("error out"=w302:errorcluster, "PhoenixMotorControlDevRef"=w301:T9)  [unwired: 9 in]
      n84 = call "Limit_Switches.vi"() -> ()  [unwired: 10 in, 2 out]
      n85 = call <vilib>:"CTRE_Phoenix_MotorControl_RefNumRegistryGet.vi"("refnum name"="Elevate") -> ("error out"=w304:errorcluster, "PhoenixMotorControlDevRef"=w303:T9)  [unwired: 9 in]
      n86 = call <vilib>:"WPI_SwitchRefNum Registry Get.vi"("refnum name"="Elevate Sensor") -> ("error out"=w310:errorcluster, "SwitchDevRef"=w309:T4)  [unwired: 9 in]
      n87 = call <vilib>:"CTRE_Phoenix_MotorControl_RefNumRegistryGet.vi"("refnum name"="Shoot") -> ("error out"=w288:errorcluster, "PhoenixMotorControlDevRef"=w287:T9)  [unwired: 9 in]
      n88 = while {
        tunnel: w310 -> [w442]
        tunnel: w309 -> [w441]
        tunnel: w308 -> [w440]
        tunnel: w307 -> [w439]
        tunnel: w306 -> [w438]
        tunnel: w305 -> [w437]
        tunnel: w304 -> [w434]
        tunnel: w303 -> [w433]
        tunnel: w302 -> [w432]
        tunnel: w301 -> [w431]
        tunnel: w300 -> [w430]
        tunnel: w299 -> [w429]
        tunnel: [w417] -> w292
        tunnel: [w416] -> w291
        tunnel: [w415] -> w290
        tunnel: [w414] -> w289
        tunnel: w288 -> [w413]
        tunnel: w287 -> [w412]
        tunnel: [w409] -> w286
        tunnel: [w408] -> w285
        tunnel: [w407] -> w278
        tunnel: [w406] -> w277
        i -> [w445]
        stop <- w446 stop-if-true
        w411 = T13 0 items=["PercentOutput"=0, "Position"=1, "Velocity"=2, "Current"=3, "Follower"=5, "MotionProfile"=6, "MotionMagic"=7, "MotionProfileArc"=10, "Disabled"=15] ("Control Mode")
        w423 = T13 0 items=["PercentOutput"=0, "Position"=1, "Velocity"=2, "Current"=3, "Follower"=5, "MotionProfile"=6, "MotionMagic"=7, "MotionProfileArc"=10, "Disabled"=15] ("Control Mode")
        w424 = T13 0 items=["PercentOutput"=0, "Position"=1, "Velocity"=2, "Current"=3, "Follower"=5, "MotionProfile"=6, "MotionMagic"=7, "MotionProfileArc"=10, "Disabled"=15] ("Control Mode")
        w425 = T13 0 items=["PercentOutput"=0, "Position"=1, "Velocity"=2, "Current"=3, "Follower"=5, "MotionProfile"=6, "MotionMagic"=7, "MotionProfileArc"=10, "Disabled"=15] ("Control Mode")
        n89 = call <vilib>:"WPI_SwitchGetLimitValue.vi"("error in (no error)"=w440, "SwitchDevRef"=w439) -> ("Switch Pressed"=w443:bool)  [unwired: 7 in, 2 out]
        n90 = call <vilib>:"WPI_SwitchGetLimitValue.vi"("error in (no error)"=w442, "SwitchDevRef"=w441) -> ("Switch Pressed"=w444:bool)  [unwired: 7 in, 2 out]
        n91 = Greater?(x=w445, y=20) -> (0:w446:bool)
        n92 = Not(x=w443) -> (.not. x?=w428:bool)
        "Intake 3" <- w428
        n93 = Not(x=w444) -> (.not. x?=w436:bool)
        "Elevate 3" <- w436
        n94 = Wait (ms)(milliseconds to wait=u32 100) -> ()  [unwired: 1 out]
        n95 = case shown="True" w436 {
          tunnel: [0.75 ("Output") w465] -> w435
          tunnel: w428 -> [_ w462]
          tunnel: [0.75 ("Output") w464] -> w427
          tunnel: [-0.1 ("Output") w463] -> w426
          tunnel: [FALSE ("Middle Thumb") w461] -> w422
          tunnel: [0.0 ("Z") w460] -> w421
          tunnel: [0.0 ("Y") w459] -> w420
          tunnel: [0.0 ("X") w458] -> w419
          tunnel: [WPI_SolenoidValue."Reverse" ("Value") w457] -> w418
          frame False {
          }
          frame True {
            n96 = case shown="False" w462 {
              tunnel: [0.75 ("Output") 0.0 ("Output")] -> w465
              tunnel: [0.75 ("Output") -0.75 ("Output")] -> w464
              tunnel: [0.0 ("Output") 0.0 ("Output")] -> w463
              tunnel: [FALSE ("Middle Thumb") FALSE ("Middle Thumb")] -> w461
              tunnel: [0.0 ("Z") 0.0 ("Z")] -> w460
              tunnel: [-0.3 ("Y") 0.0 ("Y")] -> w459
              tunnel: [0.0 ("X") 0.0 ("X")] -> w458
              tunnel: [WPI_SolenoidValue."Reverse" ("Value") WPI_SolenoidValue."Forward" ("Value")] -> w457
              frame False {
              }
              frame True {
              }
            }
          }
        }
        n97 = call-poly <vilib>:"WPI_SolenoidSet.vi"("error in (no error)"=w438, "Value"=w418, "SolenoidDevRef"=w437) -> ("error out"=w406:errorcluster, "SolenoidDevRef"=w407:T7)  [unwired: 7 in]
        n98 = call <vilib>:"CTRE_Phoenix_MotorControl_Set.vi"("error in (no error)"=w430, "Output"=w435, "Control Mode"=w423, "PhoenixMotorControlDevRef"=w429) -> ("error out"=w415:errorcluster, "PhoenixMotorControlDevRef"=w414:T9)  [unwired: 6 in]
        n99 = call <vilib>:"CTRE_Phoenix_MotorControl_Set.vi"("error in (no error)"=w432, "Output"=w427, "Control Mode"=w424, "PhoenixMotorControlDevRef"=w431) -> ()  [unwired: 6 in, 2 out]
        n100 = call <vilib>:"CTRE_Phoenix_MotorControl_Set.vi"("error in (no error)"=w434, "Output"=w426, "Control Mode"=w425, "PhoenixMotorControlDevRef"=w433) -> ("error out"=w417:errorcluster, "PhoenixMotorControlDevRef"=w416:T9)  [unwired: 6 in]
        n101 = call <vilib>:"CTRE_Phoenix_MotorControl_Set.vi"("error in (no error)"=w413, "Output"=-0.55, "Control Mode"=w411, "PhoenixMotorControlDevRef"=w412) -> ("error out"=w409:errorcluster, "PhoenixMotorControlDevRef"=w408:T9)  [unwired: 6 in]
        n102 = call "Drive_Vi.vi"("Middle Thumb"=w422, "Z"=w421, "Y"=w420, "X"=w419) -> ()  [unwired: 8 in]
      }
      n103 = call <vilib>:"WPI_SwitchRefNum Registry Get.vi"("refnum name"="Orange Limit Switch") -> ("error out"=w294:errorcluster, "SwitchDevRef"=w293:T4)  [unwired: 9 in]
      n104 = call <vilib>:"WPI_SwitchRefNum Registry Get.vi"("refnum name"="Blue Limit Switch") -> ("error out"=w296:errorcluster, "SwitchDevRef"=w295:T4)  [unwired: 9 in]
      n105 = while {
        tunnel: w286 -> [_]
        tunnel: w285 -> [_]
        tunnel: w296 -> [w403]
        tunnel: w295 -> [w402]
        tunnel: w294 -> [w401]
        tunnel: w293 -> [w400]
        tunnel: w292 -> [w379]
        tunnel: w291 -> [w378]
        tunnel: w290 -> [w369]
        tunnel: w289 -> [w370]
        tunnel: [w383] -> w284
        tunnel: [w382] -> w283
        tunnel: [w381] -> w282
        tunnel: [w380] -> w281
        tunnel: [w379] -> w280
        tunnel: [w378] -> w279
        tunnel: w278 -> [w377]
        tunnel: w277 -> [w376]
        tunnel: [w374] -> w276
        tunnel: [w373] -> w275
        tunnel: [w372] -> w274
        tunnel: [w371] -> w273
        i -> [w389]
        stop <- w388 stop-if-true
        w368 = T13 0 items=["PercentOutput"=0, "Position"=1, "Velocity"=2, "Current"=3, "Follower"=5, "MotionProfile"=6, "MotionMagic"=7, "MotionProfileArc"=10, "Disabled"=15] ("Control Mode")
        n106 = call-poly <vilib>:"WPI_SolenoidSet.vi"("error in (no error)"=w376, "Value"=WPI_SolenoidValue."Forward", "SolenoidDevRef"=w377) -> ("error out"=w373:errorcluster, "SolenoidDevRef"=w374:T7)  [unwired: 7 in]
        n107 = call <vilib>:"WPI_SwitchGetLimitValue.vi"("error in (no error)"=w401, "SwitchDevRef"=w400) -> ("error out"=w380:errorcluster, "Switch Pressed"=w399:bool, "SwitchDevRef"=w381:T4)  [unwired: 7 in]
        "Orange Limit Pressed 5" <- w399
        n108 = call <vilib>:"WPI_SwitchGetLimitValue.vi"("error in (no error)"=w403, "SwitchDevRef"=w402) -> ("error out"=w382:errorcluster, "Switch Pressed"=w398:bool, "SwitchDevRef"=w383:T4)  [unwired: 7 in]
        "Blue Limit Pressed 5" <- w398
        n109 = call-poly <vilib>:"NT Read Value.vi"("Default Value"=0.0, "Name"="/limelight-drtrain/ty") -> ("Numeric"=w393:dbl)  [unwired: 8 in, 1 out]
        "Ty 5" <- w393
        n110 = Greater?(x=w389, y=5) -> (0:w388:bool)
        n111 = call "Turret_Aim.vi"("View Button"=FALSE ("Driver Right Thumb"), "Left Trigger"=2.0, "Orange Limit Pressed"=w398, "Blue Limit Pressed"=w399, "Right Bumper"=FALSE, "Left Bumper"=FALSE) -> ()  [unwired: 6 in]
        n112 = call "Shooter_Equation.vi"("Right Trigger"=2.0, "Ty"=w393) -> ()  [unwired: 10 in]
        n113 = Wait (ms)(milliseconds to wait=u32 100) -> ()  [unwired: 1 out]
        n114 = call "Drive_Vi.vi"("Middle Thumb"=FALSE, "Z"=0.0, "Y"=0.15, "X"=0.0) -> ()  [unwired: 8 in]
        n115 = call <vilib>:"CTRE_Phoenix_MotorControl_Set.vi"("error in (no error)"=w369, "Output"=0.0, "Control Mode"=w368, "PhoenixMotorControlDevRef"=w370) -> ("error out"=w371:errorcluster, "PhoenixMotorControlDevRef"=w372:T9)  [unwired: 6 in]
      }
      n116 = while {
        tunnel: w283 -> [w364]
        tunnel: w284 -> [w363]
        tunnel: w281 -> [w362]
        tunnel: w280 -> [w349]
        tunnel: w279 -> [w348]
        tunnel: w273 -> [w347]
        tunnel: w274 -> [w346]
        tunnel: w282 -> [w337]
        tunnel: w276 -> [w336]
        tunnel: w275 -> [w335]
        tunnel: [w333] -> w272
        tunnel: [w332] -> w271
        tunnel: [w331] -> w270
        tunnel: [w330] -> w269
        i -> [w351]
        stop <- w350 stop-if-true
        w344 = T13 0 items=["PercentOutput"=0, "Position"=1, "Velocity"=2, "Current"=3, "Follower"=5, "MotionProfile"=6, "MotionMagic"=7, "MotionProfileArc"=10, "Disabled"=15] ("Control Mode")
        w345 = T13 0 items=["PercentOutput"=0, "Position"=1, "Velocity"=2, "Current"=3, "Follower"=5, "MotionProfile"=6, "MotionMagic"=7, "MotionProfileArc"=10, "Disabled"=15] ("Control Mode")
        n117 = call-poly <vilib>:"WPI_SolenoidSet.vi"("error in (no error)"=w335, "Value"=WPI_SolenoidValue."Off", "SolenoidDevRef"=w336) -> ()  [unwired: 7 in, 2 out]
        n118 = call <vilib>:"WPI_SwitchGetLimitValue.vi"("error in (no error)"=w362, "SwitchDevRef"=w337) -> ("Switch Pressed"=w361:bool)  [unwired: 7 in, 2 out]
        "Orange Limit Pressed 6" <- w361
        n119 = call <vilib>:"WPI_SwitchGetLimitValue.vi"("error in (no error)"=w364, "SwitchDevRef"=w363) -> ("Switch Pressed"=w360:bool)  [unwired: 7 in, 2 out]
        "Blue Limit Pressed 6" <- w360
        n120 = call-poly <vilib>:"NT Read Value.vi"("Default Value"=0.0, "Name"="/limelight-drtrain/ty") -> ("Numeric"=w355:dbl)  [unwired: 8 in, 1 out]
        "Ty 6" <- w355
        n121 = Greater?(x=w351, y=50) -> (0:w350:bool)
        n122 = call "Turret_Aim.vi"("View Button"=FALSE ("Driver Right Thumb"), "Left Trigger"=2.0, "Orange Limit Pressed"=w360, "Blue Limit Pressed"=w361, "Right Bumper"=FALSE, "Left Bumper"=FALSE) -> ()  [unwired: 6 in]
        n123 = call "Shooter_Equation.vi"("Right Trigger"=2.0, "Ty"=w355) -> ()  [unwired: 10 in]
        n124 = Wait (ms)(milliseconds to wait=u32 100) -> ()  [unwired: 1 out]
        n125 = call "Drive_Vi.vi"("Middle Thumb"=FALSE, "Z"=0.0, "Y"=0.15, "X"=0.0) -> ()  [unwired: 8 in]
        n126 = call <vilib>:"CTRE_Phoenix_MotorControl_Set.vi"("error in (no error)"=w347, "Output"=0.35, "Control Mode"=w344, "PhoenixMotorControlDevRef"=w346) -> ("error out"=w333:errorcluster, "PhoenixMotorControlDevRef"=w332:T9)  [unwired: 6 in]
        n127 = call <vilib>:"CTRE_Phoenix_MotorControl_Set.vi"("error in (no error)"=w349, "Output"=-0.35, "Control Mode"=w345, "PhoenixMotorControlDevRef"=w348) -> ("error out"=w330:errorcluster, "PhoenixMotorControlDevRef"=w331:T9)  [unwired: 6 in]
      }
      n128 = while {
        tunnel: w272 -> [w325]
        tunnel: w271 -> [w324]
        tunnel: w270 -> [w323]
        tunnel: w269 -> [w322]
        i -> [w320]
        stop <- w319 stop-if-true
        w328 = T13 0 items=["PercentOutput"=0, "Position"=1, "Velocity"=2, "Current"=3, "Follower"=5, "MotionProfile"=6, "MotionMagic"=7, "MotionProfileArc"=10, "Disabled"=15] ("Control Mode")
        w329 = T13 0 items=["PercentOutput"=0, "Position"=1, "Velocity"=2, "Current"=3, "Follower"=5, "MotionProfile"=6, "MotionMagic"=7, "MotionProfileArc"=10, "Disabled"=15] ("Control Mode")
        n129 = call <vilib>:"CTRE_Phoenix_MotorControl_Set.vi"("error in (no error)"=w325, "Output"=0.0, "Control Mode"=w328, "PhoenixMotorControlDevRef"=w324) -> ()  [unwired: 6 in, 2 out]
        n130 = call <vilib>:"CTRE_Phoenix_MotorControl_Set.vi"("error in (no error)"=w322, "Output"=0.0, "Control Mode"=w329, "PhoenixMotorControlDevRef"=w323) -> ()  [unwired: 6 in, 2 out]
        n131 = Greater?(x=w320, y=50) -> (0:w319:bool)
        n132 = Wait (ms)(milliseconds to wait=u32 100) -> ()  [unwired: 1 out]
      }
    }
    frame "2 Ball" {
      # "Pigeon Set"
      n133 = while {
        i -> [w699]
        stop <- w700 stop-if-true
        n134 = Wait (ms)(milliseconds to wait=u32 20) -> ()  [unwired: 1 out]
        n135 = Greater?(x=w699, y=2) -> (0:w700:bool)
        n136 = call "Drive_Vi.vi"("Middle Thumb"=TRUE, "Z"=0.0, "Y"=0.0, "X"=0.0) -> ()  [unwired: 8 in]
      }
      n137 = call <vilib>:"WPI_SwitchRefNum Registry Get.vi"("refnum name"="Intake Sensor") -> ("error out"=w528:errorcluster, "SwitchDevRef"=w527:T4)  [unwired: 9 in]
      n138 = call <vilib>:"CTRE_Phoenix_MotorControl_RefNumRegistryGet.vi"("refnum name"="Intake") -> ("error out"=w522:errorcluster, "PhoenixMotorControlDevRef"=w521:T9)  [unwired: 9 in]
      n139 = call <vilib>:"CTRE_Phoenix_MotorControl_RefNumRegistryGet.vi"("refnum name"="Intake Actuate") -> ("error out"=w493:errorcluster, "PhoenixMotorControlDevRef"=w492:T9)  [unwired: 9 in]
      n140 = call <vilib>:"CTRE_Phoenix_MotorControl_RefNumRegistryGet.vi"("refnum name"="Reject") -> ("error out"=w524:errorcluster, "PhoenixMotorControlDevRef"=w523:T9)  [unwired: 9 in]
      n141 = call "Limit_Switches.vi"() -> ()  [unwired: 10 in, 2 out]
      n142 = call <vilib>:"CTRE_Phoenix_MotorControl_RefNumRegistryGet.vi"("refnum name"="Elevate") -> ("error out"=w526:errorcluster, "PhoenixMotorControlDevRef"=w525:T9)  [unwired: 9 in]
      n143 = call <vilib>:"WPI_SwitchRefNum Registry Get.vi"("refnum name"="Elevate Sensor") -> ("error out"=w530:errorcluster, "SwitchDevRef"=w529:T4)  [unwired: 9 in]
      n144 = call <vilib>:"CTRE_Phoenix_MotorControl_RefNumRegistryGet.vi"("refnum name"="Shoot") -> ("error out"=w510:errorcluster, "PhoenixMotorControlDevRef"=w509:T9)  [unwired: 9 in]
      n145 = while {
        tunnel: w530 -> [w658]
        tunnel: w529 -> [w657]
        tunnel: w528 -> [w656]
        tunnel: w527 -> [w655]
        tunnel: w526 -> [w652]
        tunnel: w525 -> [w651]
        tunnel: w524 -> [w650]
        tunnel: w523 -> [w649]
        tunnel: w522 -> [w648]
        tunnel: w521 -> [w647]
        tunnel: [w636] -> w514
        tunnel: [w635] -> w513
        tunnel: [w634] -> w512
        tunnel: [w633] -> w511
        tunnel: w510 -> [w632]
        tunnel: w509 -> [w631]
        tunnel: [w628] -> w508
        tunnel: [w627] -> w507
        tunnel: w493 -> [w626]
        tunnel: w492 -> [w625]
        tunnel: [w622] -> w491
        tunnel: [w621] -> w490
        i -> [w661]
        stop <- w662 stop-if-true
        w624 = T13 0 items=["PercentOutput"=0, "Position"=1, "Velocity"=2, "Current"=3, "Follower"=5, "MotionProfile"=6, "MotionMagic"=7, "MotionProfileArc"=10, "Disabled"=15] ("Control Mode")
        w630 = T13 0 items=["PercentOutput"=0, "Position"=1, "Velocity"=2, "Current"=3, "Follower"=5, "MotionProfile"=6, "MotionMagic"=7, "MotionProfileArc"=10, "Disabled"=15] ("Control Mode")
        w641 = T13 0 items=["PercentOutput"=0, "Position"=1, "Velocity"=2, "Current"=3, "Follower"=5, "MotionProfile"=6, "MotionMagic"=7, "MotionProfileArc"=10, "Disabled"=15] ("Control Mode")
        w642 = T13 0 items=["PercentOutput"=0, "Position"=1, "Velocity"=2, "Current"=3, "Follower"=5, "MotionProfile"=6, "MotionMagic"=7, "MotionProfileArc"=10, "Disabled"=15] ("Control Mode")
        w643 = T13 0 items=["PercentOutput"=0, "Position"=1, "Velocity"=2, "Current"=3, "Follower"=5, "MotionProfile"=6, "MotionMagic"=7, "MotionProfileArc"=10, "Disabled"=15] ("Control Mode")
        n146 = call <vilib>:"CTRE_Phoenix_MotorControl_Set.vi"("error in (no error)"=w626, "Output"=-0.1, "Control Mode"=w624, "PhoenixMotorControlDevRef"=w625) -> ("error out"=w621:errorcluster, "PhoenixMotorControlDevRef"=w622:T9)  [unwired: 6 in]
        n147 = call <vilib>:"WPI_SwitchGetLimitValue.vi"("error in (no error)"=w656, "SwitchDevRef"=w655) -> ("Switch Pressed"=w659:bool)  [unwired: 7 in, 2 out]
        n148 = call <vilib>:"WPI_SwitchGetLimitValue.vi"("error in (no error)"=w658, "SwitchDevRef"=w657) -> ("Switch Pressed"=w660:bool)  [unwired: 7 in, 2 out]
        n149 = Greater?(x=w661, y=20) -> (0:w662:bool)
        n150 = Not(x=w659) -> (.not. x?=w646:bool)
        "Intake" <- w646
        n151 = Not(x=w660) -> (.not. x?=w654:bool)
        "Elevate" <- w654
        n152 = Wait (ms)(milliseconds to wait=u32 100) -> ()  [unwired: 1 out]
        n153 = case shown="True" w654 {
          tunnel: [0.75 ("Output") w679] -> w653
          tunnel: w646 -> [_ w676]
          tunnel: [0.75 ("Output") w678] -> w645
          tunnel: [-0.1 ("Output") w677] -> w644
          tunnel: [FALSE ("Middle Thumb") w675] -> w640
          tunnel: [0.0 ("Z") w674] -> w639
          tunnel: [0.0 ("Y") w673] -> w638
          tunnel: [0.0 ("X") w672] -> w637
          frame False {
            (unwired) WPI_SolenoidValue."Reverse" ("Value")
          }
          frame True {
            n154 = case shown="False" w676 {
              tunnel: [0.75 ("Output") 0.0 ("Output")] -> w679
              tunnel: [0.0 ("Output") 0.0 ("Output")] -> w678
              tunnel: [0.0 ("Output") 0.0 ("Output")] -> w677
              tunnel: [FALSE ("Middle Thumb") FALSE ("Middle Thumb")] -> w675
              tunnel: [0.0 ("Z") 0.0 ("Z")] -> w674
              tunnel: [-0.3 ("Y") 0.0 ("Y")] -> w673
              tunnel: [0.0 ("X") 0.0 ("X")] -> w672
              frame False {
              }
              frame True {
                (unwired) WPI_SolenoidValue."Forward" ("Value")
              }
            }
          }
        }
        n155 = call <vilib>:"CTRE_Phoenix_MotorControl_Set.vi"("error in (no error)"=w648, "Output"=w653, "Control Mode"=w641, "PhoenixMotorControlDevRef"=w647) -> ("error out"=w634:errorcluster, "PhoenixMotorControlDevRef"=w633:T9)  [unwired: 6 in]
        n156 = call <vilib>:"CTRE_Phoenix_MotorControl_Set.vi"("error in (no error)"=w650, "Output"=w645, "Control Mode"=w642, "PhoenixMotorControlDevRef"=w649) -> ()  [unwired: 6 in, 2 out]
        n157 = call <vilib>:"CTRE_Phoenix_MotorControl_Set.vi"("error in (no error)"=w652, "Output"=w644, "Control Mode"=w643, "PhoenixMotorControlDevRef"=w651) -> ("error out"=w636:errorcluster, "PhoenixMotorControlDevRef"=w635:T9)  [unwired: 6 in]
        n158 = call <vilib>:"CTRE_Phoenix_MotorControl_Set.vi"("error in (no error)"=w632, "Output"=-0.55, "Control Mode"=w630, "PhoenixMotorControlDevRef"=w631) -> ("error out"=w628:errorcluster, "PhoenixMotorControlDevRef"=w627:T9)  [unwired: 6 in]
        n159 = call "Drive_Vi.vi"("Middle Thumb"=w640, "Z"=w639, "Y"=w638, "X"=w637) -> ()  [unwired: 8 in]
      }
      n160 = call <vilib>:"WPI_SwitchRefNum Registry Get.vi"("refnum name"="Orange Limit Switch") -> ("error out"=w516:errorcluster, "SwitchDevRef"=w515:T4)  [unwired: 9 in]
      n161 = call <vilib>:"WPI_SwitchRefNum Registry Get.vi"("refnum name"="Blue Limit Switch") -> ("error out"=w518:errorcluster, "SwitchDevRef"=w517:T4)  [unwired: 9 in]
      n162 = while {
        tunnel: w508 -> [_]
        tunnel: w507 -> [_]
        tunnel: w518 -> [w618]
        tunnel: w517 -> [w617]
        tunnel: w516 -> [w616]
        tunnel: w515 -> [w615]
        tunnel: w514 -> [w594]
        tunnel: w513 -> [w593]
        tunnel: w512 -> [w589]
        tunnel: w511 -> [w590]
        tunnel: [w598] -> w506
        tunnel: [w597] -> w505
        tunnel: [w596] -> w504
        tunnel: [w595] -> w503
        tunnel: [w594] -> w502
        tunnel: [w593] -> w501
        tunnel: [w592] -> w500
        tunnel: [w591] -> w499
        tunnel: w491 -> [w584]
        tunnel: w490 -> [w583]
        i -> [w604]
        stop <- w603 stop-if-true
        w586 = T13 0 items=["PercentOutput"=0, "Position"=1, "Velocity"=2, "Current"=3, "Follower"=5, "MotionProfile"=6, "MotionMagic"=7, "MotionProfileArc"=10, "Disabled"=15] ("Control Mode")
        w588 = T13 0 items=["PercentOutput"=0, "Position"=1, "Velocity"=2, "Current"=3, "Follower"=5, "MotionProfile"=6, "MotionMagic"=7, "MotionProfileArc"=10, "Disabled"=15] ("Control Mode")
        n163 = call <vilib>:"CTRE_Phoenix_MotorControl_Set.vi"("error in (no error)"=w583, "Output"=0.0, "Control Mode"=w586, "PhoenixMotorControlDevRef"=w584) -> ()  [unwired: 6 in, 2 out]
        n164 = call <vilib>:"WPI_SwitchGetLimitValue.vi"("error in (no error)"=w616, "SwitchDevRef"=w615) -> ("error out"=w595:errorcluster, "Switch Pressed"=w614:bool, "SwitchDevRef"=w596:T4)  [unwired: 7 in]
        "Orange Limit Pressed" <- w614
        n165 = call <vilib>:"WPI_SwitchGetLimitValue.vi"("error in (no error)"=w618, "SwitchDevRef"=w617) -> ("error out"=w597:errorcluster, "Switch Pressed"=w613:bool, "SwitchDevRef"=w598:T4)  [unwired: 7 in]
        "Blue Limit Pressed" <- w613
        n166 = call-poly <vilib>:"NT Read Value.vi"("Default Value"=0.0, "Name"="/limelight-drtrain/ty") -> ("Numeric"=w608:dbl)  [unwired: 8 in, 1 out]
        "Ty" <- w608
        n167 = Greater?(x=w604, y=5) -> (0:w603:bool)
        n168 = call "Turret_Aim.vi"("View Button"=FALSE ("Driver Right Thumb"), "Left Trigger"=2.0, "Orange Limit Pressed"=w613, "Blue Limit Pressed"=w614, "Right Bumper"=FALSE, "Left Bumper"=FALSE) -> ()  [unwired: 6 in]
        n169 = call "Shooter_Equation.vi"("Right Trigger"=2.0, "Ty"=w608) -> ()  [unwired: 10 in]
        n170 = Wait (ms)(milliseconds to wait=u32 100) -> ()  [unwired: 1 out]
        n171 = call "Drive_Vi.vi"("Middle Thumb"=FALSE, "Z"=0.0, "Y"=0.15, "X"=0.0) -> ()  [unwired: 8 in]
        n172 = call <vilib>:"CTRE_Phoenix_MotorControl_Set.vi"("error in (no error)"=w589, "Output"=0.0, "Control Mode"=w588, "PhoenixMotorControlDevRef"=w590) -> ("error out"=w591:errorcluster, "PhoenixMotorControlDevRef"=w592:T9)  [unwired: 6 in]
      }
      n173 = while {
        tunnel: w505 -> [w580]
        tunnel: w506 -> [w579]
        tunnel: w503 -> [w578]
        tunnel: w502 -> [w565]
        tunnel: w501 -> [w564]
        tunnel: w499 -> [w563]
        tunnel: w500 -> [w562]
        tunnel: w504 -> [w553]
        tunnel: [w552] -> w498
        tunnel: [w551] -> w497
        tunnel: [w550] -> w496
        tunnel: [w549] -> w495
        i -> [w567]
        stop <- w566 stop-if-true
        w560 = T13 0 items=["PercentOutput"=0, "Position"=1, "Velocity"=2, "Current"=3, "Follower"=5, "MotionProfile"=6, "MotionMagic"=7, "MotionProfileArc"=10, "Disabled"=15] ("Control Mode")
        w561 = T13 0 items=["PercentOutput"=0, "Position"=1, "Velocity"=2, "Current"=3, "Follower"=5, "MotionProfile"=6, "MotionMagic"=7, "MotionProfileArc"=10, "Disabled"=15] ("Control Mode")
        n174 = call <vilib>:"WPI_SwitchGetLimitValue.vi"("error in (no error)"=w578, "SwitchDevRef"=w553) -> ("Switch Pressed"=w577:bool)  [unwired: 7 in, 2 out]
        "Orange Limit Pressed 2" <- w577
        n175 = call <vilib>:"WPI_SwitchGetLimitValue.vi"("error in (no error)"=w580, "SwitchDevRef"=w579) -> ("Switch Pressed"=w576:bool)  [unwired: 7 in, 2 out]
        "Blue Limit Pressed 2" <- w576
        n176 = call-poly <vilib>:"NT Read Value.vi"("Default Value"=0.0, "Name"="/limelight-drtrain/ty") -> ("Numeric"=w571:dbl)  [unwired: 8 in, 1 out]
        "Ty 2" <- w571
        n177 = Greater?(x=w567, y=50) -> (0:w566:bool)
        n178 = call "Turret_Aim.vi"("View Button"=FALSE ("Driver Right Thumb"), "Left Trigger"=2.0, "Orange Limit Pressed"=w576, "Blue Limit Pressed"=w577, "Right Bumper"=FALSE, "Left Bumper"=FALSE) -> ()  [unwired: 6 in]
        n179 = call "Shooter_Equation.vi"("Right Trigger"=2.0, "Ty"=w571) -> ()  [unwired: 10 in]
        n180 = Wait (ms)(milliseconds to wait=u32 100) -> ()  [unwired: 1 out]
        n181 = call "Drive_Vi.vi"("Middle Thumb"=FALSE, "Z"=0.0, "Y"=0.15, "X"=0.0) -> ()  [unwired: 8 in]
        n182 = call <vilib>:"CTRE_Phoenix_MotorControl_Set.vi"("error in (no error)"=w563, "Output"=0.35, "Control Mode"=w560, "PhoenixMotorControlDevRef"=w562) -> ("error out"=w552:errorcluster, "PhoenixMotorControlDevRef"=w551:T9)  [unwired: 6 in]
        n183 = call <vilib>:"CTRE_Phoenix_MotorControl_Set.vi"("error in (no error)"=w565, "Output"=-0.35, "Control Mode"=w561, "PhoenixMotorControlDevRef"=w564) -> ("error out"=w549:errorcluster, "PhoenixMotorControlDevRef"=w550:T9)  [unwired: 6 in]
      }
      n184 = while {
        tunnel: w498 -> [w544]
        tunnel: w497 -> [w543]
        tunnel: w496 -> [w542]
        tunnel: w495 -> [w541]
        i -> [w539]
        stop <- w538 stop-if-true
        w547 = T13 0 items=["PercentOutput"=0, "Position"=1, "Velocity"=2, "Current"=3, "Follower"=5, "MotionProfile"=6, "MotionMagic"=7, "MotionProfileArc"=10, "Disabled"=15] ("Control Mode")
        w548 = T13 0 items=["PercentOutput"=0, "Position"=1, "Velocity"=2, "Current"=3, "Follower"=5, "MotionProfile"=6, "MotionMagic"=7, "MotionProfileArc"=10, "Disabled"=15] ("Control Mode")
        n185 = call <vilib>:"CTRE_Phoenix_MotorControl_Set.vi"("error in (no error)"=w544, "Output"=0.0, "Control Mode"=w547, "PhoenixMotorControlDevRef"=w543) -> ()  [unwired: 6 in, 2 out]
        n186 = call <vilib>:"CTRE_Phoenix_MotorControl_Set.vi"("error in (no error)"=w541, "Output"=0.0, "Control Mode"=w548, "PhoenixMotorControlDevRef"=w542) -> ()  [unwired: 6 in, 2 out]
        n187 = Greater?(x=w539, y=50) -> (0:w538:bool)
        n188 = Wait (ms)(milliseconds to wait=u32 100) -> ()  [unwired: 1 out]
      }
    }
    frame "Drive Test" {
      # "Get limelight position and shooter started up"
      # "Driving backwards, put arms down and running intake to get ball"
      n189 = call <vilib>:"CTRE_Phoenix_MotorControl_RefNumRegistryGet.vi"("refnum name"="Intake") -> ("error out"=w703:errorcluster, "PhoenixMotorControlDevRef"=w705:T9)  [unwired: 9 in]
      n190 = while {
        tunnel: [w712] -> w704
        tunnel: w705 -> [w712]
        tunnel: [w711] -> w702
        tunnel: w703 -> [w711]
        i -> [w718]
        stop <- w719 stop-if-true
        n191 = Wait (ms)(milliseconds to wait=u32 20) -> ()  [unwired: 1 out]
        n192 = Greater?(x=w718, y=2) -> (0:w719:bool)
        n193 = call "Drive_Vi.vi"("Middle Thumb"=TRUE, "Z"=0.0, "Y"=0.0, "X"=0.0) -> ()  [unwired: 8 in]
      }
      n194 = while {
        tunnel: w704 -> [w752]
        tunnel: w702 -> [w751]
        tunnel: [w750] -> w709
        tunnel: [w749] -> w708
        i -> [w759]
        stop <- w758 stop-if-true
        w748 = T13 0 items=["PercentOutput"=0, "Position"=1, "Velocity"=2, "Current"=3, "Follower"=5, "MotionProfile"=6, "MotionMagic"=7, "MotionProfileArc"=10, "Disabled"=15] ("Control Mode")
        # "-0.186"
        # "-0.944"
        # ".135"
        n195 = call "Drive_Vi.vi"("Middle Thumb"=FALSE, "Z"=0.0, "Y"=-0.5, "X"=0.0) -> ()  [unwired: 8 in]
        n196 = call <vilib>:"CTRE_Phoenix_MotorControl_Set.vi"("error in (no error)"=w751, "Output"=0.0, "Control Mode"=w748, "PhoenixMotorControlDevRef"=w752) -> ("error out"=w749:errorcluster, "PhoenixMotorControlDevRef"=w750:T9)  [unwired: 6 in]
        n197 = Greater?(x=w759, y=20) -> (0:w758:bool)
        n198 = Wait (ms)(milliseconds to wait=u32 100) -> ()  [unwired: 1 out]
      }
      n199 = while {
        tunnel: w709 -> [w738]
        tunnel: w708 -> [w737]
        tunnel: [w736] -> w707
        tunnel: [w735] -> w706
        i -> [w745]
        stop <- w744 stop-if-true
        w734 = T13 0 items=["PercentOutput"=0, "Position"=1, "Velocity"=2, "Current"=3, "Follower"=5, "MotionProfile"=6, "MotionMagic"=7, "MotionProfileArc"=10, "Disabled"=15] ("Control Mode")
        # "-0.186"
        # "-0.944"
        # ".135"
        n200 = call "Drive_Vi.vi"("Middle Thumb"=FALSE, "Z"=0.0, "Y"=0.15, "X"=0.0) -> ()  [unwired: 8 in]
        n201 = Greater?(x=w745, y=5) -> (0:w744:bool)
        n202 = call <vilib>:"CTRE_Phoenix_MotorControl_Set.vi"("error in (no error)"=w737, "Output"=0.0, "Control Mode"=w734, "PhoenixMotorControlDevRef"=w738) -> ("error out"=w735:errorcluster, "PhoenixMotorControlDevRef"=w736:T9)  [unwired: 6 in]
        n203 = Wait (ms)(milliseconds to wait=u32 100) -> ()  [unwired: 1 out]
      }
      n204 = while {
        tunnel: w707 -> [w724]
        tunnel: w706 -> [w723]
        i -> [w731]
        stop <- w730 stop-if-true
        w722 = T13 0 items=["PercentOutput"=0, "Position"=1, "Velocity"=2, "Current"=3, "Follower"=5, "MotionProfile"=6, "MotionMagic"=7, "MotionProfileArc"=10, "Disabled"=15] ("Control Mode")
        # "-0.186"
        # "-0.944"
        # ".135"
        n205 = call "Drive_Vi.vi"("Middle Thumb"=FALSE, "Z"=0.0, "Y"=0.0, "X"=0.0) -> ()  [unwired: 8 in]
        n206 = Greater?(x=w731, y=20) -> (0:w730:bool)
        n207 = call <vilib>:"CTRE_Phoenix_MotorControl_Set.vi"("error in (no error)"=w723, "Output"=0.0, "Control Mode"=w722, "PhoenixMotorControlDevRef"=w724) -> ()  [unwired: 6 in, 2 out]
        n208 = Wait (ms)(milliseconds to wait=u32 100) -> ()  [unwired: 1 out]
      }
    }
    frame "4 Ball" {
      # "Pigeon Set"
      n209 = while {
        i -> [w1144]
        stop <- w1145 stop-if-true
        n210 = Wait (ms)(milliseconds to wait=u32 20) -> ()  [unwired: 1 out]
        n211 = Greater?(x=w1144, y=2) -> (0:w1145:bool)
        n212 = call "Drive_Vi.vi"("Middle Thumb"=TRUE, "Z"=0.0, "Y"=0.0, "X"=0.0) -> ()  [unwired: 8 in]
      }
      n213 = call <vilib>:"WPI_SwitchRefNum Registry Get.vi"("refnum name"="Intake Sensor") -> ("error out"=w821:errorcluster, "SwitchDevRef"=w820:T4)  [unwired: 9 in]
      n214 = call <vilib>:"CTRE_Phoenix_MotorControl_RefNumRegistryGet.vi"("refnum name"="Intake") -> ("error out"=w815:errorcluster, "PhoenixMotorControlDevRef"=w814:T9)  [unwired: 9 in]
      n215 = call <vilib>:"CTRE_Phoenix_MotorControl_RefNumRegistryGet.vi"("refnum name"="Reject") -> ("error out"=w817:errorcluster, "PhoenixMotorControlDevRef"=w816:T9)  [unwired: 9 in]
      n216 = call "Limit_Switches.vi"() -> ()  [unwired: 10 in, 2 out]
      n217 = call <vilib>:"CTRE_Phoenix_MotorControl_RefNumRegistryGet.vi"("refnum name"="Elevate") -> ("error out"=w819:errorcluster, "PhoenixMotorControlDevRef"=w818:T9)  [unwired: 9 in]
      n218 = call <vilib>:"WPI_SwitchRefNum Registry Get.vi"("refnum name"="Elevate Sensor") -> ("error out"=w823:errorcluster, "SwitchDevRef"=w822:T4)  [unwired: 9 in]
      n219 = call <vilib>:"CTRE_Phoenix_MotorControl_RefNumRegistryGet.vi"("refnum name"="Shoot") -> ("error out"=w803:errorcluster, "PhoenixMotorControlDevRef"=w802:T9)  [unwired: 9 in]
      n220 = call <vilib>:"CTRE_Phoenix_MotorControl_RefNumRegistryGet.vi"("refnum name"="Intake Actuate") -> ("error out"=w769:errorcluster, "PhoenixMotorControlDevRef"=w770:T9)  [unwired: 9 in]
      n221 = while {
        tunnel: w823 -> [w1103]
        tunnel: w822 -> [w1102]
        tunnel: w821 -> [w1101]
        tunnel: w820 -> [w1100]
        tunnel: w819 -> [w1097]
        tunnel: w818 -> [w1096]
        tunnel: w817 -> [w1095]
        tunnel: w816 -> [w1094]
        tunnel: w815 -> [w1093]
        tunnel: w814 -> [w1092]
        tunnel: [w1081] -> w807
        tunnel: [w1080] -> w806
        tunnel: [w1079] -> w805
        tunnel: [w1078] -> w804
        tunnel: w803 -> [w1077]
        tunnel: w802 -> [w1076]
        tunnel: [w1073] -> w801
        tunnel: [w1072] -> w800
        i -> [w1106]
        stop <- w1107 stop-if-true
        w1075 = T13 0 items=["PercentOutput"=0, "Position"=1, "Velocity"=2, "Current"=3, "Follower"=5, "MotionProfile"=6, "MotionMagic"=7, "MotionProfileArc"=10, "Disabled"=15] ("Control Mode")
        w1086 = T13 0 items=["PercentOutput"=0, "Position"=1, "Velocity"=2, "Current"=3, "Follower"=5, "MotionProfile"=6, "MotionMagic"=7, "MotionProfileArc"=10, "Disabled"=15] ("Control Mode")
        w1087 = T13 0 items=["PercentOutput"=0, "Position"=1, "Velocity"=2, "Current"=3, "Follower"=5, "MotionProfile"=6, "MotionMagic"=7, "MotionProfileArc"=10, "Disabled"=15] ("Control Mode")
        w1088 = T13 0 items=["PercentOutput"=0, "Position"=1, "Velocity"=2, "Current"=3, "Follower"=5, "MotionProfile"=6, "MotionMagic"=7, "MotionProfileArc"=10, "Disabled"=15] ("Control Mode")
        n222 = call <vilib>:"WPI_SwitchGetLimitValue.vi"("error in (no error)"=w1101, "SwitchDevRef"=w1100) -> ("Switch Pressed"=w1104:bool)  [unwired: 7 in, 2 out]
        n223 = call <vilib>:"WPI_SwitchGetLimitValue.vi"("error in (no error)"=w1103, "SwitchDevRef"=w1102) -> ("Switch Pressed"=w1105:bool)  [unwired: 7 in, 2 out]
        n224 = Greater?(x=w1106, y=20) -> (0:w1107:bool)
        n225 = Not(x=w1104) -> (.not. x?=w1091:bool)
        "Intake 2" <- w1091
        n226 = Not(x=w1105) -> (.not. x?=w1099:bool)
        "Elevate 2" <- w1099
        n227 = Wait (ms)(milliseconds to wait=u32 100) -> ()  [unwired: 1 out]
        n228 = case shown="True" w1099 {
          tunnel: [0.75 ("Output") w1124] -> w1098
          tunnel: w1091 -> [_ w1121]
          tunnel: [0.75 ("Output") w1123] -> w1090
          tunnel: [-0.1 ("Output") w1122] -> w1089
          tunnel: [FALSE ("Middle Thumb") w1120] -> w1085
          tunnel: [0.0 ("Z") w1119] -> w1084
          tunnel: [0.0 ("Y") w1118] -> w1083
          tunnel: [0.0 ("X") w1117] -> w1082
          frame False {
            (unwired) WPI_SolenoidValue."Reverse" ("Value")
          }
          frame True {
            n229 = case shown="False" w1121 {
              tunnel: [0.75 ("Output") 0.0 ("Output")] -> w1124
              tunnel: [0.0 ("Output") 0.0 ("Output")] -> w1123
              tunnel: [0.0 ("Output") 0.0 ("Output")] -> w1122
              tunnel: [FALSE ("Middle Thumb") FALSE ("Middle Thumb")] -> w1120
              tunnel: [0.0 ("Z") 0.0 ("Z")] -> w1119
              tunnel: [-0.3 ("Y") 0.0 ("Y")] -> w1118
              tunnel: [0.0 ("X") 0.0 ("X")] -> w1117
              frame False {
              }
              frame True {
                (unwired) WPI_SolenoidValue."Forward" ("Value")
              }
            }
          }
        }
        n230 = call <vilib>:"CTRE_Phoenix_MotorControl_Set.vi"("error in (no error)"=w1093, "Output"=w1098, "Control Mode"=w1086, "PhoenixMotorControlDevRef"=w1092) -> ("error out"=w1079:errorcluster, "PhoenixMotorControlDevRef"=w1078:T9)  [unwired: 6 in]
        n231 = call <vilib>:"CTRE_Phoenix_MotorControl_Set.vi"("error in (no error)"=w1095, "Output"=w1090, "Control Mode"=w1087, "PhoenixMotorControlDevRef"=w1094) -> ()  [unwired: 6 in, 2 out]
        n232 = call <vilib>:"CTRE_Phoenix_MotorControl_Set.vi"("error in (no error)"=w1097, "Output"=w1089, "Control Mode"=w1088, "PhoenixMotorControlDevRef"=w1096) -> ("error out"=w1081:errorcluster, "PhoenixMotorControlDevRef"=w1080:T9)  [unwired: 6 in]
        n233 = call <vilib>:"CTRE_Phoenix_MotorControl_Set.vi"("error in (no error)"=w1077, "Output"=-0.55, "Control Mode"=w1075, "PhoenixMotorControlDevRef"=w1076) -> ("error out"=w1073:errorcluster, "PhoenixMotorControlDevRef"=w1072:T9)  [unwired: 6 in]
        n234 = call "Drive_Vi.vi"("Middle Thumb"=w1085, "Z"=w1084, "Y"=w1083, "X"=w1082) -> ()  [unwired: 8 in]
      }
      n235 = while {
        tunnel: w770 -> [w851]
        tunnel: w769 -> [w850]
        i -> [w843]
        stop <- w842 stop-if-true
        n236 = for {
          N: 20 -> [_]
          tunnel: w851 -> [w863]
          tunnel: w850 -> [w862]
          tunnel: [w861] -> w849 mode=indexing
          tunnel: [w860] -> w848 mode=indexing
          w858 = T13 0 items=["PercentOutput"=0, "Position"=1, "Velocity"=2, "Current"=3, "Follower"=5, "MotionProfile"=6, "MotionMagic"=7, "MotionProfileArc"=10, "Disabled"=15] ("Control Mode")
          n237 = call <vilib>:"CTRE_Phoenix_MotorControl_Set.vi"("error in (no error)"=w862, "Output"=-0.1, "Control Mode"=w858, "PhoenixMotorControlDevRef"=w863) -> ("error out"=w860:errorcluster, "PhoenixMotorControlDevRef"=w861:T9)  [unwired: 6 in]
          n238 = Wait (ms)(milliseconds to wait=u32 35) -> ()  [unwired: 1 out]
        }
        n239 = for {
          N: 20 -> [_]
          tunnel: w849 -> [w856] mode=indexing
          tunnel: w848 -> [w855] mode=indexing
          w853 = T13 0 items=["PercentOutput"=0, "Position"=1, "Velocity"=2, "Current"=3, "Follower"=5, "MotionProfile"=6, "MotionMagic"=7, "MotionProfileArc"=10, "Disabled"=15] ("Control Mode")
          n240 = Wait (ms)(milliseconds to wait=u32 50) -> ()  [unwired: 1 out]
          n241 = call <vilib>:"CTRE_Phoenix_MotorControl_Set.vi"("error in (no error)"=w855, "Output"=0.0, "Control Mode"=w853, "PhoenixMotorControlDevRef"=w856) -> ()  [unwired: 6 in, 2 out]
        }
        n242 = Greater?(x=w843, y=2) -> (0:w842:bool)
        n243 = Wait (ms)(milliseconds to wait=u32 20) -> ()  [unwired: 1 out]
      }
      n244 = call <vilib>:"WPI_SwitchRefNum Registry Get.vi"("refnum name"="Orange Limit Switch") -> ("error out"=w809:errorcluster, "SwitchDevRef"=w808:T4)  [unwired: 9 in]
      n245 = call <vilib>:"WPI_SwitchRefNum Registry Get.vi"("refnum name"="Blue Limit Switch") -> ("error out"=w811:errorcluster, "SwitchDevRef"=w810:T4)  [unwired: 9 in]
      n246 = while {
        tunnel: w801 -> [_]
        tunnel: w800 -> [_]
        tunnel: w811 -> [w1069]
        tunnel: w810 -> [w1068]
        tunnel: w809 -> [w1067]
        tunnel: w808 -> [w1066]
        tunnel: w807 -> [w1045]
        tunnel: w806 -> [w1044]
        tunnel: w805 -> [w1040]
        tunnel: w804 -> [w1041]
        tunnel: [w1049] -> w799
        tunnel: [w1048] -> w798
        tunnel: [w1047] -> w797
        tunnel: [w1046] -> w796
        tunnel: [w1045] -> w795
        tunnel: [w1044] -> w794
        tunnel: [w1043] -> w793
        tunnel: [w1042] -> w792
        i -> [w1055]
        stop <- w1054 stop-if-true
        w1039 = T13 0 items=["PercentOutput"=0, "Position"=1, "Velocity"=2, "Current"=3, "Follower"=5, "MotionProfile"=6, "MotionMagic"=7, "MotionProfileArc"=10, "Disabled"=15] ("Control Mode")
        n247 = call <vilib>:"WPI_SwitchGetLimitValue.vi"("error in (no error)"=w1067, "SwitchDevRef"=w1066) -> ("error out"=w1046:errorcluster, "Switch Pressed"=w1065:bool, "SwitchDevRef"=w1047:T4)  [unwired: 7 in]
        "Orange Limit Pressed 3" <- w1065
        n248 = call <vilib>:"WPI_SwitchGetLimitValue.vi"("error in (no error)"=w1069, "SwitchDevRef"=w1068) -> ("error out"=w1048:errorcluster, "Switch Pressed"=w1064:bool, "SwitchDevRef"=w1049:T4)  [unwired: 7 in]
        "Blue Limit Pressed 3" <- w1064
        n249 = call-poly <vilib>:"NT Read Value.vi"("Default Value"=0.0, "Name"="/limelight-drtrain/ty") -> ("Numeric"=w1059:dbl)  [unwired: 8 in, 1 out]
        "Ty 3" <- w1059
        n250 = Greater?(x=w1055, y=5) -> (0:w1054:bool)
        n251 = call "Turret_Aim.vi"("View Button"=FALSE ("Driver Right Thumb"), "Left Trigger"=2.0, "Orange Limit Pressed"=w1064, "Blue Limit Pressed"=w1065, "Right Bumper"=FALSE, "Left Bumper"=FALSE) -> ()  [unwired: 6 in]
        n252 = call "Shooter_Equation.vi"("Right Trigger"=2.0, "Ty"=w1059) -> ()  [unwired: 10 in]
        n253 = Wait (ms)(milliseconds to wait=u32 100) -> ()  [unwired: 1 out]
        n254 = call "Drive_Vi.vi"("Middle Thumb"=FALSE, "Z"=0.0, "Y"=0.15, "X"=0.0) -> ()  [unwired: 8 in]
        n255 = call <vilib>:"CTRE_Phoenix_MotorControl_Set.vi"("error in (no error)"=w1040, "Output"=0.0, "Control Mode"=w1039, "PhoenixMotorControlDevRef"=w1041) -> ("error out"=w1042:errorcluster, "PhoenixMotorControlDevRef"=w1043:T9)  [unwired: 6 in]
      }
      n256 = while {
        tunnel: w798 -> [w1035]
        tunnel: w799 -> [w1034]
        tunnel: w796 -> [w1033]
        tunnel: w795 -> [w1020]
        tunnel: w794 -> [w1019]
        tunnel: w792 -> [w1018]
        tunnel: w793 -> [w1017]
        tunnel: w797 -> [w1008]
        tunnel: [w1007] -> w791
        tunnel: [w1006] -> w790
        tunnel: [w1005] -> w789
        tunnel: [w1004] -> w788
        i -> [w1022]
        stop <- w1021 stop-if-true
        w1015 = T13 0 items=["PercentOutput"=0, "Position"=1, "Velocity"=2, "Current"=3, "Follower"=5, "MotionProfile"=6, "MotionMagic"=7, "MotionProfileArc"=10, "Disabled"=15] ("Control Mode")
        w1016 = T13 0 items=["PercentOutput"=0, "Position"=1, "Velocity"=2, "Current"=3, "Follower"=5, "MotionProfile"=6, "MotionMagic"=7, "MotionProfileArc"=10, "Disabled"=15] ("Control Mode")
        # "40"
        n257 = call <vilib>:"WPI_SwitchGetLimitValue.vi"("error in (no error)"=w1033, "SwitchDevRef"=w1008) -> ("Switch Pressed"=w1032:bool)  [unwired: 7 in, 2 out]
        "Orange Limit Pressed 4" <- w1032
        n258 = call <vilib>:"WPI_SwitchGetLimitValue.vi"("error in (no error)"=w1035, "SwitchDevRef"=w1034) -> ("Switch Pressed"=w1031:bool)  [unwired: 7 in, 2 out]
        "Blue Limit Pressed 4" <- w1031
        n259 = call-poly <vilib>:"NT Read Value.vi"("Default Value"=0.0, "Name"="/limelight-drtrain/ty") -> ("Numeric"=w1026:dbl)  [unwired: 8 in, 1 out]
        "Ty 4" <- w1026
        n260 = Greater?(x=w1022, y=20) -> (0:w1021:bool)
        n261 = call "Turret_Aim.vi"("View Button"=FALSE ("Driver Right Thumb"), "Left Trigger"=2.0, "Orange Limit Pressed"=w1031, "Blue Limit Pressed"=w1032, "Right Bumper"=FALSE, "Left Bumper"=FALSE) -> ()  [unwired: 6 in]
        n262 = call "Shooter_Equation.vi"("Right Trigger"=2.0, "Ty"=w1026) -> ()  [unwired: 10 in]
        n263 = Wait (ms)(milliseconds to wait=u32 100) -> ()  [unwired: 1 out]
        n264 = call "Drive_Vi.vi"("Middle Thumb"=FALSE, "Z"=0.0, "Y"=0.15, "X"=0.0) -> ()  [unwired: 8 in]
        n265 = call <vilib>:"CTRE_Phoenix_MotorControl_Set.vi"("error in (no error)"=w1018, "Output"=0.35, "Control Mode"=w1015, "PhoenixMotorControlDevRef"=w1017) -> ("error out"=w1007:errorcluster, "PhoenixMotorControlDevRef"=w1006:T9)  [unwired: 6 in]
        n266 = call <vilib>:"CTRE_Phoenix_MotorControl_Set.vi"("error in (no error)"=w1020, "Output"=-0.35, "Control Mode"=w1016, "PhoenixMotorControlDevRef"=w1019) -> ("error out"=w1004:errorcluster, "PhoenixMotorControlDevRef"=w1005:T9)  [unwired: 6 in]
      }
      n267 = while {
        tunnel: w791 -> [w999]
        tunnel: w790 -> [w998]
        tunnel: w789 -> [w997]
        tunnel: w788 -> [w996]
        tunnel: [w987] -> w768
        tunnel: [w986] -> w766
        tunnel: [w985] -> w764
        tunnel: [w984] -> w762
        i -> [w994]
        stop <- w993 stop-if-true
        w1002 = T13 0 items=["PercentOutput"=0, "Position"=1, "Velocity"=2, "Current"=3, "Follower"=5, "MotionProfile"=6, "MotionMagic"=7, "MotionProfileArc"=10, "Disabled"=15] ("Control Mode")
        w1003 = T13 0 items=["PercentOutput"=0, "Position"=1, "Velocity"=2, "Current"=3, "Follower"=5, "MotionProfile"=6, "MotionMagic"=7, "MotionProfileArc"=10, "Disabled"=15] ("Control Mode")
        n268 = call <vilib>:"CTRE_Phoenix_MotorControl_Set.vi"("error in (no error)"=w999, "Output"=0.0, "Control Mode"=w1002, "PhoenixMotorControlDevRef"=w998) -> ("error out"=w986:errorcluster, "PhoenixMotorControlDevRef"=w987:T9)  [unwired: 6 in]
        n269 = call <vilib>:"CTRE_Phoenix_MotorControl_Set.vi"("error in (no error)"=w996, "Output"=0.0, "Control Mode"=w1003, "PhoenixMotorControlDevRef"=w997) -> ("error out"=w984:errorcluster, "PhoenixMotorControlDevRef"=w985:T9)  [unwired: 6 in]
        n270 = call "Drive_Vi.vi"("Middle Thumb"=FALSE, "Z"=-0.35, "Y"=0.0, "X"=0.0) -> ()  [unwired: 8 in]
        n271 = Greater?(x=w994, y=5) -> (0:w993:bool)
        n272 = Wait (ms)(milliseconds to wait=u32 100) -> ()  [unwired: 1 out]
        n273 = call-poly <vilib>:"NT Read Value.vi"("Default Value"=0.0, "Name"="/limelight-drtrain/ty") -> ("Numeric"=w989:dbl)  [unwired: 8 in, 1 out]
        "Ty 9" <- w989
        n274 = call "Shooter_Equation.vi"("Right Trigger"=0.0, "Ty"=w989) -> ()  [unwired: 10 in]
      }
      n275 = while {
        tunnel: [w833] -> w767
        tunnel: w768 -> [w833]
        tunnel: [w832] -> w765
        tunnel: w766 -> [w832]
        tunnel: [w831] -> w763
        tunnel: w764 -> [w831]
        tunnel: [w830] -> w761
        tunnel: w762 -> [w830]
        i -> [w839]
        stop <- w840 stop-if-true
        n276 = Wait (ms)(milliseconds to wait=u32 20) -> ()  [unwired: 1 out]
        n277 = Greater?(x=w839, y=5) -> (0:w840:bool)
        n278 = call "Drive_Vi.vi"("Middle Thumb"=TRUE, "Z"=0.0, "Y"=0.0, "X"=0.0) -> ()  [unwired: 8 in]
      }
      n279 = while {
        tunnel: w767 -> [w963]
        tunnel: w765 -> [w962]
        tunnel: w763 -> [w961]
        tunnel: w761 -> [w960]
        tunnel: [w959] -> w787
        tunnel: [w958] -> w786
        tunnel: [w957] -> w785
        tunnel: [w956] -> w784
        i -> [w974]
        stop <- w973 stop-if-true
        w978 = T13 0 items=["PercentOutput"=0, "Position"=1, "Velocity"=2, "Current"=3, "Follower"=5, "MotionProfile"=6, "MotionMagic"=7, "MotionProfileArc"=10, "Disabled"=15] ("Control Mode")
        w979 = T13 0 items=["PercentOutput"=0, "Position"=1, "Velocity"=2, "Current"=3, "Follower"=5, "MotionProfile"=6, "MotionMagic"=7, "MotionProfileArc"=10, "Disabled"=15] ("Control Mode")
        # "-0.186"
        # "-0.944"
        # ".135"
        n280 = call "Drive_Vi.vi"("Middle Thumb"=FALSE, "Z"=0.0, "Y"=-0.8, "X"=0.0) -> ()  [unwired: 8 in]
        n281 = call <vilib>:"CTRE_Phoenix_MotorControl_Set.vi"("error in (no error)"=w962, "Output"=0.0, "Control Mode"=w978, "PhoenixMotorControlDevRef"=w963) -> ("error out"=w958:errorcluster, "PhoenixMotorControlDevRef"=w959:T9)  [unwired: 6 in]
        n282 = call <vilib>:"CTRE_Phoenix_MotorControl_Set.vi"("error in (no error)"=w960, "Output"=0.0, "Control Mode"=w979, "PhoenixMotorControlDevRef"=w961) -> ("error out"=w956:errorcluster, "PhoenixMotorControlDevRef"=w957:T9)  [unwired: 6 in]
        n283 = Greater?(x=w974, y=8) -> (0:w973:bool)
        n284 = Wait (ms)(milliseconds to wait=u32 100) -> ()  [unwired: 1 out]
        n285 = call-poly <vilib>:"NT Read Value.vi"("Default Value"=0.0, "Name"="/limelight-drtrain/ty") -> ("Numeric"=w965:dbl)  [unwired: 8 in, 1 out]
        "Ty 10" <- w965
        n286 = call "Shooter_Equation.vi"("Right Trigger"=0.0, "Ty"=w965) -> ()  [unwired: 10 in]
      }
      n287 = while {
        tunnel: w787 -> [w947]
        tunnel: w786 -> [w946]
        tunnel: w785 -> [w945]
        tunnel: w784 -> [w944]
        tunnel: [w939] -> w783
        tunnel: [w938] -> w782
        tunnel: [w937] -> w781
        tunnel: [w936] -> w780
        i -> [w941]
        stop <- w940 stop-if-true
        w954 = T13 0 items=["PercentOutput"=0, "Position"=1, "Velocity"=2, "Current"=3, "Follower"=5, "MotionProfile"=6, "MotionMagic"=7, "MotionProfileArc"=10, "Disabled"=15] ("Control Mode")
        w955 = T13 0 items=["PercentOutput"=0, "Position"=1, "Velocity"=2, "Current"=3, "Follower"=5, "MotionProfile"=6, "MotionMagic"=7, "MotionProfileArc"=10, "Disabled"=15] ("Control Mode")
        # "-0.186"
        # "-0.944"
        # ".135"
        n288 = call <vilib>:"CTRE_Phoenix_MotorControl_Set.vi"("error in (no error)"=w946, "Output"=0.0, "Control Mode"=w954, "PhoenixMotorControlDevRef"=w947) -> ("error out"=w938:errorcluster, "PhoenixMotorControlDevRef"=w939:T9)  [unwired: 6 in]
        n289 = call <vilib>:"CTRE_Phoenix_MotorControl_Set.vi"("error in (no error)"=w944, "Output"=0.0, "Control Mode"=w955, "PhoenixMotorControlDevRef"=w945) -> ("error out"=w936:errorcluster, "PhoenixMotorControlDevRef"=w937:T9)  [unwired: 6 in]
        n290 = call "Drive_Vi.vi"("Middle Thumb"=FALSE, "Z"=0.0, "Y"=0.0, "X"=0.0) -> ()  [unwired: 8 in]
        n291 = Greater?(x=w941, y=5) -> (0:w940:bool)
        n292 = call-poly <vilib>:"NT Read Value.vi"("Default Value"=0.0, "Name"="/limelight-drtrain/ty") -> ("Numeric"=w949:dbl)  [unwired: 8 in, 1 out]
        "Ty 11" <- w949
        n293 = Wait (ms)(milliseconds to wait=u32 100) -> ()  [unwired: 1 out]
        n294 = call "Shooter_Equation.vi"("Right Trigger"=0.0, "Ty"=w949) -> ()  [unwired: 10 in]
      }
      n295 = while {
        tunnel: w783 -> [w919]
        tunnel: w782 -> [w918]
        tunnel: w781 -> [w917]
        tunnel: w780 -> [w916]
        tunnel: [w911] -> w779
        tunnel: [w910] -> w778
        tunnel: [w909] -> w777
        tunnel: [w908] -> w776
        i -> [w913]
        stop <- w912 stop-if-true
        w930 = T13 0 items=["PercentOutput"=0, "Position"=1, "Velocity"=2, "Current"=3, "Follower"=5, "MotionProfile"=6, "MotionMagic"=7, "MotionProfileArc"=10, "Disabled"=15] ("Control Mode")
        w931 = T13 0 items=["PercentOutput"=0, "Position"=1, "Velocity"=2, "Current"=3, "Follower"=5, "MotionProfile"=6, "MotionMagic"=7, "MotionProfileArc"=10, "Disabled"=15] ("Control Mode")
        # "-0.186"
        # "-0.944"
        # ".135"
        n296 = call "Drive_Vi.vi"("Middle Thumb"=FALSE, "Z"=0.0, "Y"=0.0, "X"=0.0) -> ()  [unwired: 8 in]
        n297 = call <vilib>:"CTRE_Phoenix_MotorControl_Set.vi"("error in (no error)"=w918, "Output"=0.75, "Control Mode"=w930, "PhoenixMotorControlDevRef"=w919) -> ("error out"=w910:errorcluster, "PhoenixMotorControlDevRef"=w911:T9)  [unwired: 6 in]
        n298 = call <vilib>:"CTRE_Phoenix_MotorControl_Set.vi"("error in (no error)"=w916, "Output"=-0.1, "Control Mode"=w931, "PhoenixMotorControlDevRef"=w917) -> ("error out"=w908:errorcluster, "PhoenixMotorControlDevRef"=w909:T9)  [unwired: 6 in]
        n299 = Greater?(x=w913, y=20) -> (0:w912:bool)
        n300 = Wait (ms)(milliseconds to wait=u32 100) -> ()  [unwired: 1 out]
        n301 = call-poly <vilib>:"NT Read Value.vi"("Default Value"=0.0, "Name"="/limelight-drtrain/ty") -> ("Numeric"=w921:dbl)  [unwired: 8 in, 1 out]
        "Ty 12" <- w921
        n302 = call "Shooter_Equation.vi"("Right Trigger"=0.0, "Ty"=w921) -> ()  [unwired: 10 in]
      }
      n303 = while {
        tunnel: w779 -> [w895]
        tunnel: [w888] -> _
        tunnel: w777 -> [w894]
        tunnel: w776 -> [w893]
        tunnel: w778 -> [w888]
        tunnel: [w887] -> w775
        tunnel: [w886] -> w774
        tunnel: [w885] -> w773
        tunnel: [w884] -> w772
        i -> [w890]
        stop <- w889 stop-if-true
        w906 = T13 0 items=["PercentOutput"=0, "Position"=1, "Velocity"=2, "Current"=3, "Follower"=5, "MotionProfile"=6, "MotionMagic"=7, "MotionProfileArc"=10, "Disabled"=15] ("Control Mode")
        w907 = T13 0 items=["PercentOutput"=0, "Position"=1, "Velocity"=2, "Current"=3, "Follower"=5, "MotionProfile"=6, "MotionMagic"=7, "MotionProfileArc"=10, "Disabled"=15] ("Control Mode")
        # "-0.186"
        # "-0.944"
        # ".135"
        n304 = call "Drive_Vi.vi"("Middle Thumb"=FALSE, "Z"=0.0, "Y"=0.0, "X"=0.0) -> ()  [unwired: 8 in]
        n305 = call <vilib>:"CTRE_Phoenix_MotorControl_Set.vi"("error in (no error)"=w888, "Output"=0.0, "Control Mode"=w906, "PhoenixMotorControlDevRef"=w895) -> ("error out"=w884:errorcluster, "PhoenixMotorControlDevRef"=w885:T9)  [unwired: 6 in]
        n306 = call <vilib>:"CTRE_Phoenix_MotorControl_Set.vi"("error in (no error)"=w893, "Output"=0.0, "Control Mode"=w907, "PhoenixMotorControlDevRef"=w894) -> ("error out"=w887:errorcluster, "PhoenixMotorControlDevRef"=w886:T9)  [unwired: 6 in]
        n307 = Greater?(x=w890, y=10) -> (0:w889:bool)
        n308 = Wait (ms)(milliseconds to wait=u32 100) -> ()  [unwired: 1 out]
        n309 = call-poly <vilib>:"NT Read Value.vi"("Default Value"=0.0, "Name"="/limelight-drtrain/ty") -> ("Numeric"=w897:dbl)  [unwired: 8 in, 1 out]
        "Ty 13" <- w897
        n310 = call "Shooter_Equation.vi"("Right Trigger"=0.0, "Ty"=w897) -> ()  [unwired: 10 in]
      }
      n311 = while {
        tunnel: w773 -> [w871]
        tunnel: [w864] -> _
        tunnel: w774 -> [w870]
        tunnel: w775 -> [w869]
        tunnel: w772 -> [w864]
        i -> [w866]
        stop <- w865 stop-if-true
        w882 = T13 0 items=["PercentOutput"=0, "Position"=1, "Velocity"=2, "Current"=3, "Follower"=5, "MotionProfile"=6, "MotionMagic"=7, "MotionProfileArc"=10, "Disabled"=15] ("Control Mode")
        w883 = T13 0 items=["PercentOutput"=0, "Position"=1, "Velocity"=2, "Current"=3, "Follower"=5, "MotionProfile"=6, "MotionMagic"=7, "MotionProfileArc"=10, "Disabled"=15] ("Control Mode")
        # "-0.186"
        # "-0.944"
        # ".135"
        n312 = call "Drive_Vi.vi"("Middle Thumb"=FALSE, "Z"=0.0, "Y"=0.0, "X"=0.0) -> ()  [unwired: 8 in]
        n313 = call <vilib>:"CTRE_Phoenix_MotorControl_Set.vi"("error in (no error)"=w864, "Output"=0.0, "Control Mode"=w882, "PhoenixMotorControlDevRef"=w871) -> ()  [unwired: 6 in, 2 out]
        n314 = call <vilib>:"CTRE_Phoenix_MotorControl_Set.vi"("error in (no error)"=w869, "Output"=0.0, "Control Mode"=w883, "PhoenixMotorControlDevRef"=w870) -> ()  [unwired: 6 in, 2 out]
        n315 = Greater?(x=w866, y=20) -> (0:w865:bool)
        n316 = Wait (ms)(milliseconds to wait=u32 100) -> ()  [unwired: 1 out]
        n317 = call-poly <vilib>:"NT Read Value.vi"("Default Value"=0.0, "Name"="/limelight-drtrain/ty") -> ("Numeric"=w873:dbl)  [unwired: 8 in, 1 out]
        "Ty 14" <- w873
        n318 = call "Shooter_Equation.vi"("Right Trigger"=0.0, "Ty"=w873) -> ()  [unwired: 10 in]
      }
    }
    frame "4 Ball Pos 3" {
      # "Pigeon Set"
      n319 = while {
        i -> [w1562]
        stop <- w1563 stop-if-true
        n320 = Wait (ms)(milliseconds to wait=u32 20) -> ()  [unwired: 1 out]
        n321 = Greater?(x=w1562, y=2) -> (0:w1563:bool)
        n322 = call "Drive_Vi.vi"("Middle Thumb"=TRUE, "Z"=0.0, "Y"=0.0, "X"=0.0) -> ()  [unwired: 8 in]
      }
      n323 = call <vilib>:"WPI_SwitchRefNum Registry Get.vi"("refnum name"="Intake Sensor") -> ("error out"=w1215:errorcluster, "SwitchDevRef"=w1214:T4)  [unwired: 9 in]
      n324 = call <vilib>:"CTRE_Phoenix_MotorControl_RefNumRegistryGet.vi"("refnum name"="Intake") -> ("error out"=w1209:errorcluster, "PhoenixMotorControlDevRef"=w1208:T9)  [unwired: 9 in]
      n325 = call <vilib>:"CTRE_Phoenix_MotorControl_RefNumRegistryGet.vi"("refnum name"="Reject") -> ("error out"=w1211:errorcluster, "PhoenixMotorControlDevRef"=w1210:T9)  [unwired: 9 in]
      n326 = call "Limit_Switches.vi"() -> ()  [unwired: 10 in, 2 out]
      n327 = call <vilib>:"CTRE_Phoenix_MotorControl_RefNumRegistryGet.vi"("refnum name"="Elevate") -> ("error out"=w1213:errorcluster, "PhoenixMotorControlDevRef"=w1212:T9)  [unwired: 9 in]
      n328 = call <vilib>:"WPI_SwitchRefNum Registry Get.vi"("refnum name"="Elevate Sensor") -> ("error out"=w1217:errorcluster, "SwitchDevRef"=w1216:T4)  [unwired: 9 in]
      n329 = call <vilib>:"CTRE_Phoenix_MotorControl_RefNumRegistryGet.vi"("refnum name"="Shoot") -> ("error out"=w1197:errorcluster, "PhoenixMotorControlDevRef"=w1196:T9)  [unwired: 9 in]
      n330 = call <vilib>:"CTRE_Phoenix_MotorControl_RefNumRegistryGet.vi"("refnum name"="Intake Actuate") -> ("error out"=w1167:errorcluster, "PhoenixMotorControlDevRef"=w1168:T9)  [unwired: 9 in]
      n331 = while {
        tunnel: w1217 -> [w1521]
        tunnel: w1216 -> [w1520]
        tunnel: w1215 -> [w1519]
        tunnel: w1214 -> [w1518]
        tunnel: w1213 -> [w1515]
        tunnel: w1212 -> [w1514]
        tunnel: w1211 -> [w1513]
        tunnel: w1210 -> [w1512]
        tunnel: w1209 -> [w1511]
        tunnel: w1208 -> [w1510]
        tunnel: [w1499] -> w1201
        tunnel: [w1498] -> w1200
        tunnel: [w1497] -> w1199
        tunnel: [w1496] -> w1198
        tunnel: w1197 -> [w1495]
        tunnel: w1196 -> [w1494]
        tunnel: [w1491] -> w1195
        tunnel: [w1490] -> w1194
        i -> [w1524]
        stop <- w1525 stop-if-true
        w1493 = T13 0 items=["PercentOutput"=0, "Position"=1, "Velocity"=2, "Current"=3, "Follower"=5, "MotionProfile"=6, "MotionMagic"=7, "MotionProfileArc"=10, "Disabled"=15] ("Control Mode")
        w1504 = T13 0 items=["PercentOutput"=0, "Position"=1, "Velocity"=2, "Current"=3, "Follower"=5, "MotionProfile"=6, "MotionMagic"=7, "MotionProfileArc"=10, "Disabled"=15] ("Control Mode")
        w1505 = T13 0 items=["PercentOutput"=0, "Position"=1, "Velocity"=2, "Current"=3, "Follower"=5, "MotionProfile"=6, "MotionMagic"=7, "MotionProfileArc"=10, "Disabled"=15] ("Control Mode")
        w1506 = T13 0 items=["PercentOutput"=0, "Position"=1, "Velocity"=2, "Current"=3, "Follower"=5, "MotionProfile"=6, "MotionMagic"=7, "MotionProfileArc"=10, "Disabled"=15] ("Control Mode")
        n332 = call <vilib>:"WPI_SwitchGetLimitValue.vi"("error in (no error)"=w1519, "SwitchDevRef"=w1518) -> ("Switch Pressed"=w1522:bool)  [unwired: 7 in, 2 out]
        n333 = call <vilib>:"WPI_SwitchGetLimitValue.vi"("error in (no error)"=w1521, "SwitchDevRef"=w1520) -> ("Switch Pressed"=w1523:bool)  [unwired: 7 in, 2 out]
        n334 = Greater?(x=w1524, y=20) -> (0:w1525:bool)
        n335 = Not(x=w1522) -> (.not. x?=w1509:bool)
        "Intake 5" <- w1509
        n336 = Not(x=w1523) -> (.not. x?=w1517:bool)
        "Elevate 5" <- w1517
        n337 = Wait (ms)(milliseconds to wait=u32 100) -> ()  [unwired: 1 out]
        n338 = case shown="True" w1517 {
          tunnel: [0.75 ("Output") w1542] -> w1516
          tunnel: w1509 -> [_ w1539]
          tunnel: [0.75 ("Output") w1541] -> w1508
          tunnel: [-0.1 ("Output") w1540] -> w1507
          tunnel: [FALSE ("Middle Thumb") w1538] -> w1503
          tunnel: [0.0 ("Z") w1537] -> w1502
          tunnel: [0.0 ("Y") w1536] -> w1501
          tunnel: [0.0 ("X") w1535] -> w1500
          frame False {
            (unwired) WPI_SolenoidValue."Reverse" ("Value")
          }
          frame True {
            n339 = case shown="True" w1539 {
              tunnel: [0.75 ("Output") 0.0 ("Output")] -> w1542
              tunnel: [0.0 ("Output") 0.0 ("Output")] -> w1541
              tunnel: [0.0 ("Output") 0.0 ("Output")] -> w1540
              tunnel: [FALSE ("Middle Thumb") FALSE ("Middle Thumb")] -> w1538
              tunnel: [0.0 ("Z") 0.0 ("Z")] -> w1537
              tunnel: [-0.3 ("Y") 0.0 ("Y")] -> w1536
              tunnel: [0.0 ("X") 0.0 ("X")] -> w1535
              frame False {
              }
              frame True {
              }
            }
          }
        }
        n340 = call <vilib>:"CTRE_Phoenix_MotorControl_Set.vi"("error in (no error)"=w1511, "Output"=w1516, "Control Mode"=w1504, "PhoenixMotorControlDevRef"=w1510) -> ("error out"=w1497:errorcluster, "PhoenixMotorControlDevRef"=w1496:T9)  [unwired: 6 in]
        n341 = call <vilib>:"CTRE_Phoenix_MotorControl_Set.vi"("error in (no error)"=w1513, "Output"=w1508, "Control Mode"=w1505, "PhoenixMotorControlDevRef"=w1512) -> ()  [unwired: 6 in, 2 out]
        n342 = call <vilib>:"CTRE_Phoenix_MotorControl_Set.vi"("error in (no error)"=w1515, "Output"=w1507, "Control Mode"=w1506, "PhoenixMotorControlDevRef"=w1514) -> ("error out"=w1499:errorcluster, "PhoenixMotorControlDevRef"=w1498:T9)  [unwired: 6 in]
        n343 = call <vilib>:"CTRE_Phoenix_MotorControl_Set.vi"("error in (no error)"=w1495, "Output"=-0.55, "Control Mode"=w1493, "PhoenixMotorControlDevRef"=w1494) -> ("error out"=w1491:errorcluster, "PhoenixMotorControlDevRef"=w1490:T9)  [unwired: 6 in]
        n344 = call "Drive_Vi.vi"("Middle Thumb"=w1503, "Z"=w1502, "Y"=w1501, "X"=w1500) -> ()  [unwired: 8 in]
      }
      n345 = while {
        tunnel: w1168 -> [w1257]
        tunnel: w1167 -> [w1256]
        i -> [w1249]
        stop <- w1248 stop-if-true
        n346 = for {
          N: 20 -> [_]
          tunnel: w1257 -> [w1269]
          tunnel: w1256 -> [w1268]
          tunnel: [w1267] -> w1255 mode=indexing
          tunnel: [w1266] -> w1254 mode=indexing
          w1264 = T13 0 items=["PercentOutput"=0, "Position"=1, "Velocity"=2, "Current"=3, "Follower"=5, "MotionProfile"=6, "MotionMagic"=7, "MotionProfileArc"=10, "Disabled"=15] ("Control Mode")
          n347 = call <vilib>:"CTRE_Phoenix_MotorControl_Set.vi"("error in (no error)"=w1268, "Output"=-0.1, "Control Mode"=w1264, "PhoenixMotorControlDevRef"=w1269) -> ("error out"=w1266:errorcluster, "PhoenixMotorControlDevRef"=w1267:T9)  [unwired: 6 in]
          n348 = Wait (ms)(milliseconds to wait=u32 35) -> ()  [unwired: 1 out]
        }
        n349 = for {
          N: 20 -> [_]
          tunnel: w1255 -> [w1262] mode=indexing
          tunnel: w1254 -> [w1261] mode=indexing
          w1259 = T13 0 items=["PercentOutput"=0, "Position"=1, "Velocity"=2, "Current"=3, "Follower"=5, "MotionProfile"=6, "MotionMagic"=7, "MotionProfileArc"=10, "Disabled"=15] ("Control Mode")
          n350 = Wait (ms)(milliseconds to wait=u32 50) -> ()  [unwired: 1 out]
          n351 = call <vilib>:"CTRE_Phoenix_MotorControl_Set.vi"("error in (no error)"=w1261, "Output"=0.0, "Control Mode"=w1259, "PhoenixMotorControlDevRef"=w1262) -> ()  [unwired: 6 in, 2 out]
        }
        n352 = Greater?(x=w1249, y=2) -> (0:w1248:bool)
        n353 = Wait (ms)(milliseconds to wait=u32 20) -> ()  [unwired: 1 out]
      }
      n354 = call <vilib>:"WPI_SwitchRefNum Registry Get.vi"("refnum name"="Orange Limit Switch") -> ("error out"=w1203:errorcluster, "SwitchDevRef"=w1202:T4)  [unwired: 9 in]
      n355 = call <vilib>:"WPI_SwitchRefNum Registry Get.vi"("refnum name"="Blue Limit Switch") -> ("error out"=w1205:errorcluster, "SwitchDevRef"=w1204:T4)  [unwired: 9 in]
      n356 = while {
        tunnel: w1195 -> [_]
        tunnel: w1194 -> [_]
        tunnel: w1205 -> [w1487]
        tunnel: w1204 -> [w1486]
        tunnel: w1203 -> [w1485]
        tunnel: w1202 -> [w1484]
        tunnel: w1201 -> [w1463]
        tunnel: w1200 -> [w1462]
        tunnel: w1199 -> [w1458]
        tunnel: w1198 -> [w1459]
        tunnel: [w1467] -> w1193
        tunnel: [w1466] -> w1192
        tunnel: [w1465] -> w1191
        tunnel: [w1464] -> w1190
        tunnel: [w1463] -> w1189
        tunnel: [w1462] -> w1188
        tunnel: [w1461] -> w1187
        tunnel: [w1460] -> w1186
        i -> [w1473]
        stop <- w1472 stop-if-true
        w1457 = T13 0 items=["PercentOutput"=0, "Position"=1, "Velocity"=2, "Current"=3, "Follower"=5, "MotionProfile"=6, "MotionMagic"=7, "MotionProfileArc"=10, "Disabled"=15] ("Control Mode")
        n357 = call <vilib>:"WPI_SwitchGetLimitValue.vi"("error in (no error)"=w1485, "SwitchDevRef"=w1484) -> ("error out"=w1464:errorcluster, "Switch Pressed"=w1483:bool, "SwitchDevRef"=w1465:T4)  [unwired: 7 in]
        "Orange Limit Pressed 9" <- w1483
        n358 = call <vilib>:"WPI_SwitchGetLimitValue.vi"("error in (no error)"=w1487, "SwitchDevRef"=w1486) -> ("error out"=w1466:errorcluster, "Switch Pressed"=w1482:bool, "SwitchDevRef"=w1467:T4)  [unwired: 7 in]
        "Blue Limit Pressed 9" <- w1482
        n359 = call-poly <vilib>:"NT Read Value.vi"("Default Value"=0.0, "Name"="/limelight-drtrain/ty") -> ("Numeric"=w1477:dbl)  [unwired: 8 in, 1 out]
        "Ty 15" <- w1477
        n360 = Greater?(x=w1473, y=5) -> (0:w1472:bool)
        n361 = call "Turret_Aim.vi"("View Button"=FALSE ("Driver Right Thumb"), "Left Trigger"=2.0, "Orange Limit Pressed"=w1482, "Blue Limit Pressed"=w1483, "Right Bumper"=FALSE, "Left Bumper"=FALSE) -> ()  [unwired: 6 in]
        n362 = call "Shooter_Equation.vi"("Right Trigger"=2.0, "Ty"=w1477) -> ()  [unwired: 10 in]
        n363 = Wait (ms)(milliseconds to wait=u32 100) -> ()  [unwired: 1 out]
        n364 = call "Drive_Vi.vi"("Middle Thumb"=FALSE, "Z"=0.0, "Y"=0.15, "X"=0.0) -> ()  [unwired: 8 in]
        n365 = call <vilib>:"CTRE_Phoenix_MotorControl_Set.vi"("error in (no error)"=w1458, "Output"=0.0, "Control Mode"=w1457, "PhoenixMotorControlDevRef"=w1459) -> ("error out"=w1460:errorcluster, "PhoenixMotorControlDevRef"=w1461:T9)  [unwired: 6 in]
      }
      n366 = while {
        tunnel: w1192 -> [w1453]
        tunnel: w1193 -> [w1452]
        tunnel: w1190 -> [w1451]
        tunnel: w1189 -> [w1440]
        tunnel: w1188 -> [w1439]
        tunnel: w1186 -> [w1438]
        tunnel: w1187 -> [w1437]
        tunnel: w1191 -> [w1428]
        tunnel: [w1427] -> w1185
        tunnel: [w1426] -> w1184
        tunnel: [w1425] -> w1183
        tunnel: [w1424] -> w1182
        tunnel: [w1423] -> w1150
        tunnel: [w1422] -> w1149
        i -> [w1442]
        stop <- w1441 stop-if-true
        w1435 = T13 0 items=["PercentOutput"=0, "Position"=1, "Velocity"=2, "Current"=3, "Follower"=5, "MotionProfile"=6, "MotionMagic"=7, "MotionProfileArc"=10, "Disabled"=15] ("Control Mode")
        w1436 = T13 0 items=["PercentOutput"=0, "Position"=1, "Velocity"=2, "Current"=3, "Follower"=5, "MotionProfile"=6, "MotionMagic"=7, "MotionProfileArc"=10, "Disabled"=15] ("Control Mode")
        # "40"
        n367 = call <vilib>:"WPI_SwitchGetLimitValue.vi"("error in (no error)"=w1451, "SwitchDevRef"=w1428) -> ("Switch Pressed"=w1423:bool)  [unwired: 7 in, 2 out]
        "Orange Limit Pressed 10" <- w1423
        n368 = call <vilib>:"WPI_SwitchGetLimitValue.vi"("error in (no error)"=w1453, "SwitchDevRef"=w1452) -> ("Switch Pressed"=w1422:bool)  [unwired: 7 in, 2 out]
        "Blue Limit Pressed 10" <- w1422
        n369 = call-poly <vilib>:"NT Read Value.vi"("Default Value"=0.0, "Name"="/limelight-drtrain/ty") -> ("Numeric"=w1446:dbl)  [unwired: 8 in, 1 out]
        "Ty 16" <- w1446
        n370 = Greater?(x=w1442, y=20) -> (0:w1441:bool)
        n371 = call "Turret_Aim.vi"("View Button"=FALSE ("Driver Right Thumb"), "Left Trigger"=2.0, "Orange Limit Pressed"=w1422, "Blue Limit Pressed"=w1423, "Right Bumper"=FALSE, "Left Bumper"=FALSE) -> ()  [unwired: 6 in]
        n372 = call "Shooter_Equation.vi"("Right Trigger"=2.0, "Ty"=w1446) -> ()  [unwired: 10 in]
        n373 = Wait (ms)(milliseconds to wait=u32 100) -> ()  [unwired: 1 out]
        n374 = call "Drive_Vi.vi"("Middle Thumb"=FALSE, "Z"=0.0, "Y"=0.15, "X"=0.0) -> ()  [unwired: 8 in]
        n375 = call <vilib>:"CTRE_Phoenix_MotorControl_Set.vi"("error in (no error)"=w1438, "Output"=0.35, "Control Mode"=w1435, "PhoenixMotorControlDevRef"=w1437) -> ("error out"=w1427:errorcluster, "PhoenixMotorControlDevRef"=w1426:T9)  [unwired: 6 in]
        n376 = call <vilib>:"CTRE_Phoenix_MotorControl_Set.vi"("error in (no error)"=w1440, "Output"=-0.35, "Control Mode"=w1436, "PhoenixMotorControlDevRef"=w1439) -> ("error out"=w1424:errorcluster, "PhoenixMotorControlDevRef"=w1425:T9)  [unwired: 6 in]
      }
      n377 = while {
        tunnel: w1185 -> [w1417]
        tunnel: w1184 -> [w1416]
        tunnel: w1183 -> [w1415]
        tunnel: w1182 -> [w1414]
        tunnel: [w1405] -> w1166
        tunnel: [w1404] -> w1164
        tunnel: [w1403] -> w1162
        tunnel: [w1402] -> w1160
        i -> [w1412]
        stop <- w1411 stop-if-true
        w1420 = T13 0 items=["PercentOutput"=0, "Position"=1, "Velocity"=2, "Current"=3, "Follower"=5, "MotionProfile"=6, "MotionMagic"=7, "MotionProfileArc"=10, "Disabled"=15] ("Control Mode")
        w1421 = T13 0 items=["PercentOutput"=0, "Position"=1, "Velocity"=2, "Current"=3, "Follower"=5, "MotionProfile"=6, "MotionMagic"=7, "MotionProfileArc"=10, "Disabled"=15] ("Control Mode")
        n378 = call <vilib>:"CTRE_Phoenix_MotorControl_Set.vi"("error in (no error)"=w1417, "Output"=0.0, "Control Mode"=w1420, "PhoenixMotorControlDevRef"=w1416) -> ("error out"=w1404:errorcluster, "PhoenixMotorControlDevRef"=w1405:T9)  [unwired: 6 in]
        n379 = call <vilib>:"CTRE_Phoenix_MotorControl_Set.vi"("error in (no error)"=w1414, "Output"=0.0, "Control Mode"=w1421, "PhoenixMotorControlDevRef"=w1415) -> ("error out"=w1402:errorcluster, "PhoenixMotorControlDevRef"=w1403:T9)  [unwired: 6 in]
        n380 = call "Drive_Vi.vi"("Middle Thumb"=FALSE, "Z"=0.22, "Y"=0.0, "X"=0.0) -> ()  [unwired: 8 in]
        n381 = Greater?(x=w1412, y=4) -> (0:w1411:bool)
        n382 = Wait (ms)(milliseconds to wait=u32 100) -> ()  [unwired: 1 out]
        n383 = call-poly <vilib>:"NT Read Value.vi"("Default Value"=0.0, "Name"="/limelight-drtrain/ty") -> ("Numeric"=w1407:dbl)  [unwired: 8 in, 1 out]
        "Ty 17" <- w1407
        n384 = call "Shooter_Equation.vi"("Right Trigger"=0.0, "Ty"=w1407) -> ()  [unwired: 10 in]
      }
      n385 = while {
        tunnel: [w1239] -> w1165
        tunnel: w1166 -> [w1239]
        tunnel: [w1238] -> w1163
        tunnel: w1164 -> [w1238]
        tunnel: [w1237] -> w1161
        tunnel: w1162 -> [w1237]
        tunnel: [w1236] -> w1159
        tunnel: w1160 -> [w1236]
        i -> [w1245]
        stop <- w1246 stop-if-true
        n386 = Wait (ms)(milliseconds to wait=u32 20) -> ()  [unwired: 1 out]
        n387 = Greater?(x=w1245, y=5) -> (0:w1246:bool)
        n388 = call "Drive_Vi.vi"("Middle Thumb"=TRUE, "Z"=0.0, "Y"=0.0, "X"=0.0) -> ()  [unwired: 8 in]
      }
      n389 = while {
        tunnel: w1165 -> [w1381]
        tunnel: w1163 -> [w1380]
        tunnel: w1161 -> [w1379]
        tunnel: w1159 -> [w1378]
        tunnel: [w1377] -> w1181
        tunnel: [w1376] -> w1180
        tunnel: [w1375] -> w1179
        tunnel: [w1374] -> w1178
        i -> [w1392]
        stop <- w1391 stop-if-true
        w1396 = T13 0 items=["PercentOutput"=0, "Position"=1, "Velocity"=2, "Current"=3, "Follower"=5, "MotionProfile"=6, "MotionMagic"=7, "MotionProfileArc"=10, "Disabled"=15] ("Control Mode")
        w1397 = T13 0 items=["PercentOutput"=0, "Position"=1, "Velocity"=2, "Current"=3, "Follower"=5, "MotionProfile"=6, "MotionMagic"=7, "MotionProfileArc"=10, "Disabled"=15] ("Control Mode")
        # "-0.186"
        # "-0.944"
        # ".135"
        n390 = call "Drive_Vi.vi"("Middle Thumb"=FALSE, "Z"=0.0, "Y"=-0.75, "X"=0.0) -> ()  [unwired: 8 in]
        n391 = call <vilib>:"CTRE_Phoenix_MotorControl_Set.vi"("error in (no error)"=w1380, "Output"=1.0, "Control Mode"=w1396, "PhoenixMotorControlDevRef"=w1381) -> ("error out"=w1376:errorcluster, "PhoenixMotorControlDevRef"=w1377:T9)  [unwired: 6 in]
        n392 = call <vilib>:"CTRE_Phoenix_MotorControl_Set.vi"("error in (no error)"=w1378, "Output"=0.0, "Control Mode"=w1397, "PhoenixMotorControlDevRef"=w1379) -> ("error out"=w1374:errorcluster, "PhoenixMotorControlDevRef"=w1375:T9)  [unwired: 6 in]
        n393 = Greater?(x=w1392, y=3) -> (0:w1391:bool)
        n394 = Wait (ms)(milliseconds to wait=u32 116) -> ()  [unwired: 1 out]
        n395 = call-poly <vilib>:"NT Read Value.vi"("Default Value"=0.0, "Name"="/limelight-drtrain/ty") -> ("Numeric"=w1383:dbl)  [unwired: 8 in, 1 out]
        "Ty 18" <- w1383
        n396 = call "Shooter_Equation.vi"("Right Trigger"=0.0, "Ty"=w1383) -> ()  [unwired: 10 in]
      }
      n397 = while {
        tunnel: w1181 -> [w1365]
        tunnel: w1180 -> [w1364]
        tunnel: w1179 -> [w1363]
        tunnel: w1178 -> [w1362]
        tunnel: [w1357] -> w1177
        tunnel: [w1356] -> w1176
        tunnel: [w1355] -> w1175
        tunnel: [w1354] -> w1174
        i -> [w1359]
        stop <- w1358 stop-if-true
        w1372 = T13 0 items=["PercentOutput"=0, "Position"=1, "Velocity"=2, "Current"=3, "Follower"=5, "MotionProfile"=6, "MotionMagic"=7, "MotionProfileArc"=10, "Disabled"=15] ("Control Mode")
        w1373 = T13 0 items=["PercentOutput"=0, "Position"=1, "Velocity"=2, "Current"=3, "Follower"=5, "MotionProfile"=6, "MotionMagic"=7, "MotionProfileArc"=10, "Disabled"=15] ("Control Mode")
        # "-0.186"
        # "-0.944"
        # ".135"
        n398 = call <vilib>:"CTRE_Phoenix_MotorControl_Set.vi"("error in (no error)"=w1364, "Output"=1.0, "Control Mode"=w1372, "PhoenixMotorControlDevRef"=w1365) -> ("error out"=w1356:errorcluster, "PhoenixMotorControlDevRef"=w1357:T9)  [unwired: 6 in]
        n399 = call <vilib>:"CTRE_Phoenix_MotorControl_Set.vi"("error in (no error)"=w1362, "Output"=0.0, "Control Mode"=w1373, "PhoenixMotorControlDevRef"=w1363) -> ("error out"=w1354:errorcluster, "PhoenixMotorControlDevRef"=w1355:T9)  [unwired: 6 in]
        n400 = call "Drive_Vi.vi"("Middle Thumb"=FALSE, "Z"=0.0, "Y"=0.0, "X"=0.0) -> ()  [unwired: 8 in]
        n401 = Greater?(x=w1359, y=35) -> (0:w1358:bool)
        n402 = call-poly <vilib>:"NT Read Value.vi"("Default Value"=0.0, "Name"="/limelight-drtrain/ty") -> ("Numeric"=w1367:dbl)  [unwired: 8 in, 1 out]
        "Ty 19" <- w1367
        n403 = Wait (ms)(milliseconds to wait=u32 100) -> ()  [unwired: 1 out]
        n404 = call "Shooter_Equation.vi"("Right Trigger"=0.0, "Ty"=w1367) -> ()  [unwired: 10 in]
      }
      n405 = while {
        tunnel: w1177 -> [w1337]
        tunnel: w1176 -> [w1336]
        tunnel: w1175 -> [w1335]
        tunnel: w1174 -> [w1334]
        tunnel: [w1329] -> w1173
        tunnel: [w1328] -> w1172
        tunnel: [w1327] -> w1171
        tunnel: [w1326] -> w1170
        tunnel: w1150 -> [w1320]
        tunnel: w1149 -> [w1321]
        tunnel: [w1321] -> w1148
        tunnel: [w1320] -> w1147
        i -> [w1331]
        stop <- w1330 stop-if-true
        w1348 = T13 0 items=["PercentOutput"=0, "Position"=1, "Velocity"=2, "Current"=3, "Follower"=5, "MotionProfile"=6, "MotionMagic"=7, "MotionProfileArc"=10, "Disabled"=15] ("Control Mode")
        w1349 = T13 0 items=["PercentOutput"=0, "Position"=1, "Velocity"=2, "Current"=3, "Follower"=5, "MotionProfile"=6, "MotionMagic"=7, "MotionProfileArc"=10, "Disabled"=15] ("Control Mode")
        # "-0.186"
        # "-0.944"
        # ".135"
        n406 = call "Turret_Aim.vi"("View Button"=FALSE, "Left Trigger"=0.0, "Orange Limit Pressed"=w1320, "Blue Limit Pressed"=w1321, "Right Bumper"=FALSE, "Left Bumper"=FALSE) -> ()  [unwired: 6 in]
        n407 = call "Drive_Vi.vi"("Middle Thumb"=FALSE, "Z"=0.0, "Y"=0.75, "X"=0.0) -> ()  [unwired: 8 in]
        n408 = call <vilib>:"CTRE_Phoenix_MotorControl_Set.vi"("error in (no error)"=w1336, "Output"=1.0, "Control Mode"=w1348, "PhoenixMotorControlDevRef"=w1337) -> ("error out"=w1328:errorcluster, "PhoenixMotorControlDevRef"=w1329:T9)  [unwired: 6 in]
        n409 = call <vilib>:"CTRE_Phoenix_MotorControl_Set.vi"("error in (no error)"=w1334, "Output"=-0.1, "Control Mode"=w1349, "PhoenixMotorControlDevRef"=w1335) -> ("error out"=w1326:errorcluster, "PhoenixMotorControlDevRef"=w1327:T9)  [unwired: 6 in]
        n410 = Greater?(x=w1331, y=5) -> (0:w1330:bool)
        n411 = Wait (ms)(milliseconds to wait=u32 50) -> ()  [unwired: 1 out]
        n412 = call-poly <vilib>:"NT Read Value.vi"("Default Value"=0.0, "Name"="/limelight-drtrain/ty") -> ("Numeric"=w1339:dbl)  [unwired: 8 in, 1 out]
        "Ty 20" <- w1339
        n413 = call "Shooter_Equation.vi"("Right Trigger"=0.0, "Ty"=w1339) -> ()  [unwired: 10 in]
      }
      n414 = while {
        tunnel: w1173 -> [w1307]
        tunnel: [w1300] -> _
        tunnel: w1171 -> [w1306]
        tunnel: w1170 -> [w1305]
        tunnel: w1172 -> [w1300]
        tunnel: [w1299] -> w1153
        tunnel: [w1298] -> w1152
        tunnel: [w1297] -> w1158
        tunnel: [w1296] -> w1156
        tunnel: w1148 -> [w1292]
        tunnel: w1147 -> [w1291]
        i -> [w1302]
        stop <- w1301 stop-if-true
        (unwired) FALSE ("Orange Limit Pressed")
        w1318 = T13 0 items=["PercentOutput"=0, "Position"=1, "Velocity"=2, "Current"=3, "Follower"=5, "MotionProfile"=6, "MotionMagic"=7, "MotionProfileArc"=10, "Disabled"=15] ("Control Mode")
        w1319 = T13 0 items=["PercentOutput"=0, "Position"=1, "Velocity"=2, "Current"=3, "Follower"=5, "MotionProfile"=6, "MotionMagic"=7, "MotionProfileArc"=10, "Disabled"=15] ("Control Mode")
        # "-0.186"
        # "-0.944"
        # ".135"
        n415 = call "Turret_Aim.vi"("View Button"=FALSE, "Left Trigger"=2.0, "Orange Limit Pressed"=w1291, "Blue Limit Pressed"=w1292, "Right Bumper"=FALSE, "Left Bumper"=FALSE) -> ()  [unwired: 6 in]
        n416 = call "Drive_Vi.vi"("Middle Thumb"=FALSE, "Z"=0.0, "Y"=-0.1, "X"=0.0) -> ()  [unwired: 8 in]
        n417 = call <vilib>:"CTRE_Phoenix_MotorControl_Set.vi"("error in (no error)"=w1300, "Output"=0.0, "Control Mode"=w1318, "PhoenixMotorControlDevRef"=w1307) -> ("error out"=w1296:errorcluster, "PhoenixMotorControlDevRef"=w1297:T9)  [unwired: 6 in]
        n418 = call <vilib>:"CTRE_Phoenix_MotorControl_Set.vi"("error in (no error)"=w1305, "Output"=-0.35, "Control Mode"=w1319, "PhoenixMotorControlDevRef"=w1306) -> ("error out"=w1299:errorcluster, "PhoenixMotorControlDevRef"=w1298:T9)  [unwired: 6 in]
        n419 = Greater?(x=w1302, y=10) -> (0:w1301:bool)
        n420 = Wait (ms)(milliseconds to wait=u32 100) -> ()  [unwired: 1 out]
        n421 = call-poly <vilib>:"NT Read Value.vi"("Default Value"=0.0, "Name"="/limelight-drtrain/ty") -> ("Numeric"=w1309:dbl)  [unwired: 8 in, 1 out]
        "Ty 21" <- w1309
        n422 = call "Shooter_Equation.vi"("Right Trigger"=2.0, "Ty"=w1309) -> ()  [unwired: 10 in]
      }
      n423 = while {
        tunnel: [w1235] -> w1157
        tunnel: w1158 -> [w1235]
        tunnel: [w1234] -> w1155
        tunnel: w1156 -> [w1234]
        tunnel: [w1233] -> w1154
        tunnel: w1153 -> [w1233]
        tunnel: [w1232] -> w1151
        tunnel: w1152 -> [w1232]
        i -> [w1225]
        stop <- w1224 stop-if-true
        n424 = Greater?(x=w1225, y=4) -> (0:w1224:bool)
        n425 = call "Drive_Vi.vi"("Middle Thumb"=TRUE, "Z"=0.15, "Y"=0.0, "X"=0.0) -> ()  [unwired: 8 in]
        n426 = Wait (ms)(milliseconds to wait=u32 100) -> ()  [unwired: 1 out]
      }
      n427 = while {
        tunnel: w1157 -> [w1277]
        tunnel: w1155 -> [w1270]
        tunnel: w1151 -> [w1276]
        tunnel: w1154 -> [w1275]
        i -> [w1272]
        stop <- w1271 stop-if-true
        w1288 = T13 0 items=["PercentOutput"=0, "Position"=1, "Velocity"=2, "Current"=3, "Follower"=5, "MotionProfile"=6, "MotionMagic"=7, "MotionProfileArc"=10, "Disabled"=15] ("Control Mode")
        w1289 = T13 0 items=["PercentOutput"=0, "Position"=1, "Velocity"=2, "Current"=3, "Follower"=5, "MotionProfile"=6, "MotionMagic"=7, "MotionProfileArc"=10, "Disabled"=15] ("Control Mode")
        # "-0.186"
        # "-0.944"
        # ".135"
        n428 = call "Drive_Vi.vi"("Middle Thumb"=FALSE, "Z"=0.0, "Y"=0.0, "X"=0.0) -> ()  [unwired: 8 in]
        n429 = call <vilib>:"CTRE_Phoenix_MotorControl_Set.vi"("error in (no error)"=w1270, "Output"=0.0, "Control Mode"=w1288, "PhoenixMotorControlDevRef"=w1277) -> ()  [unwired: 6 in, 2 out]
        n430 = call <vilib>:"CTRE_Phoenix_MotorControl_Set.vi"("error in (no error)"=w1275, "Output"=0.0, "Control Mode"=w1289, "PhoenixMotorControlDevRef"=w1276) -> ()  [unwired: 6 in, 2 out]
        n431 = Greater?(x=w1272, y=20) -> (0:w1271:bool)
        n432 = Wait (ms)(milliseconds to wait=u32 100) -> ()  [unwired: 1 out]
        n433 = call-poly <vilib>:"NT Read Value.vi"("Default Value"=0.0, "Name"="/limelight-drtrain/ty") -> ("Numeric"=w1279:dbl)  [unwired: 8 in, 1 out]
        "Ty 22" <- w1279
        n434 = call "Shooter_Equation.vi"("Right Trigger"=0.0, "Ty"=w1279) -> ()  [unwired: 10 in]
      }
    }
    frame "Angle Test" {
      n435 = call <vilib>:"CTRE_Phoenix_MotorControl_RefNumRegistryGet.vi"("refnum name"="Orange Back Turn") -> ("error out"=w1577:errorcluster, "PhoenixMotorControlDevRef"=w1578:T9)  [unwired: 9 in]
      n436 = call <vilib>:"CTRE_Phoenix_MotorControl_RefNumRegistryGet.vi"("refnum name"="Orange Back Drive") -> ("error out"=w1575:errorcluster, "PhoenixMotorControlDevRef"=w1576:T9)  [unwired: 9 in]
      n437 = while {
        tunnel: w1578 -> [w1621]
        tunnel: w1577 -> [w1619]
        tunnel: w1576 -> [w1614]
        tunnel: w1575 -> [w1613]
        tunnel: [w1610] -> w1572
        tunnel: [w1609] -> w1571
        tunnel: [w1608] -> w1570
        tunnel: [w1607] -> w1569
        i -> [w1624]
        stop <- w1622 stop-if-true
        w1611 = T13 0 items=["PercentOutput"=0, "Position"=1, "Velocity"=2, "Current"=3, "Follower"=5, "MotionProfile"=6, "MotionMagic"=7, "MotionProfileArc"=10, "Disabled"=15] ("Control Mode")
        w1616 = T13 0 items=["PercentOutput"=0, "Position"=1, "Velocity"=2, "Current"=3, "Follower"=5, "MotionProfile"=6, "MotionMagic"=7, "MotionProfileArc"=10, "Disabled"=15] ("Control Mode")
        n438 = call <vilib>:"CTRE_Phoenix_MotorControl_SetSelectedSensorPosition.vi"("error in (no error)"=w1619, "New Sensor Position"=0, "PhoenixMotorControlDevRef"=w1621) -> ("error out"=w1618:errorcluster, "PhoenixMotorControlDevRef"=w1620:T9)  [unwired: 7 in]
        n439 = Wait (ms)(milliseconds to wait=u32 20) -> ()  [unwired: 1 out]
        n440 = call <vilib>:"CTRE_Phoenix_MotorControl_Set.vi"("error in (no error)"=w1613, "Output"=0.0, "Control Mode"=w1611, "PhoenixMotorControlDevRef"=w1614) -> ("error out"=w1607:errorcluster, "PhoenixMotorControlDevRef"=w1608:T9)  [unwired: 6 in]
        n441 = call <vilib>:"CTRE_Phoenix_MotorControl_Set.vi"("error in (no error)"=w1618, "Output"=0.0, "Control Mode"=w1616, "PhoenixMotorControlDevRef"=w1620) -> ("error out"=w1609:errorcluster, "PhoenixMotorControlDevRef"=w1610:T9)  [unwired: 6 in]
        n442 = Greater?(x=w1624, y=u32 10) -> (0:w1622:bool)
      }
      n443 = while {
        tunnel: w1572 -> [w1595]
        tunnel: w1571 -> [w1596]
        tunnel: w1570 -> [w1600]
        tunnel: w1569 -> [w1599]
        tunnel: [w1594] -> w1568
        tunnel: [w1593] -> w1567
        tunnel: [w1592] -> w1566
        tunnel: [w1591] -> w1565
        i -> [w1605]
        stop <- w1603 stop-if-true
        w1597 = T13 0 items=["PercentOutput"=0, "Position"=1, "Velocity"=2, "Current"=3, "Follower"=5, "MotionProfile"=6, "MotionMagic"=7, "MotionProfileArc"=10, "Disabled"=15] ("Control Mode")
        w1602 = T13 1 items=["PercentOutput"=0, "Position"=1, "Velocity"=2, "Current"=3, "Follower"=5, "MotionProfile"=6, "MotionMagic"=7, "MotionProfileArc"=10, "Disabled"=15] ("Control Mode")
        n444 = Wait (ms)(milliseconds to wait=u32 20) -> ()  [unwired: 1 out]
        n445 = call <vilib>:"CTRE_Phoenix_MotorControl_Set.vi"("error in (no error)"=w1599, "Output"=0.0, "Control Mode"=w1597, "PhoenixMotorControlDevRef"=w1600) -> ("error out"=w1591:errorcluster, "PhoenixMotorControlDevRef"=w1592:T9)  [unwired: 6 in]
        n446 = call <vilib>:"CTRE_Phoenix_MotorControl_Set.vi"("error in (no error)"=w1596, "Output"=1024.0, "Control Mode"=w1602, "PhoenixMotorControlDevRef"=w1595) -> ("error out"=w1593:errorcluster, "PhoenixMotorControlDevRef"=w1594:T9)  [unwired: 6 in]
        n447 = Greater?(x=w1605, y=u32 10) -> (0:w1603:bool)
      }
      n448 = while {
        tunnel: w1568 -> [w1579]
        tunnel: w1567 -> [w1580]
        tunnel: w1566 -> [w1584]
        tunnel: w1565 -> [w1583]
        i -> [w1589]
        stop <- w1587 stop-if-true
        w1581 = T13 0 items=["PercentOutput"=0, "Position"=1, "Velocity"=2, "Current"=3, "Follower"=5, "MotionProfile"=6, "MotionMagic"=7, "MotionProfileArc"=10, "Disabled"=15] ("Control Mode")
        w1586 = T13 0 items=["PercentOutput"=0, "Position"=1, "Velocity"=2, "Current"=3, "Follower"=5, "MotionProfile"=6, "MotionMagic"=7, "MotionProfileArc"=10, "Disabled"=15] ("Control Mode")
        n449 = Wait (ms)(milliseconds to wait=u32 20) -> ()  [unwired: 1 out]
        n450 = call <vilib>:"CTRE_Phoenix_MotorControl_Set.vi"("error in (no error)"=w1583, "Output"=-0.1, "Control Mode"=w1581, "PhoenixMotorControlDevRef"=w1584) -> ()  [unwired: 6 in, 2 out]
        n451 = call <vilib>:"CTRE_Phoenix_MotorControl_Set.vi"("error in (no error)"=w1580, "Output"=0.0, "Control Mode"=w1586, "PhoenixMotorControlDevRef"=w1579) -> ()  [unwired: 6 in, 2 out]
        n452 = Greater?(x=w1589, y=u32 10) -> (0:w1587:bool)
      }
    }
  }
